vi "Read Logs.vi"() -> ()   [LabVIEW 2020]
panel:
  in  "Voltage Godograph Range":dbl caption="Amplitude Range, V" min=1.0 max=1000.0 step=1.0
  in  "Current Godograph Range":dbl caption="Amplitude Range, A" min=1.0 max=200.0 step=1.0
  in  "Voltage Amplitude Range":dbl caption="Amplitude Range, V" min=1.0 max=1000.0 step=1.0
  in  "Current Amplitude Range":dbl caption="Amplitude Range, A" min=1.0 max=200.0 step=1.0
  in  "Level Lower Limit, Cur":dbl caption="Level Lower Limit, dB" min=-200.0 max=-10.0 step=10.0
  in  "Freq Lower Limit, Cur":dbl caption="Freq Lower Limit, Hz" min=0.0 step=1.0
  in  "Freq Upper Limit, Cur":dbl caption="Freq Upper Limit, Hz" min=0.0 step=1.0
  out "Current Godograph store":cluster{"Y":dbl[], "Y":dbl[]}[](array[cluster])
  out "Voltage Godograph store":cluster{"Y":dbl[], "Y":dbl[]}[](array[cluster])
  out "Current Park Spectrum store":waveform(dbl)[](array[waveform])
  out "Voltage Park Spectrum store":waveform(dbl)[](array[waveform])
  out "Current Spectrum store":waveform(dbl)[](array[waveform])
  out "Voltage Spectrum store":waveform(dbl)[](array[waveform])
  out "Voltage store":waveform(dbl)[](array[waveform])
  out "Current store":waveform(dbl)[](array[waveform])
  in  "Hold":bool
  in  "Plot Selector":u16(ring) items=["Current", "Voltage", "Current Godograph", "Voltage Godograph", "Current Spectrum", "Voltage Spectrum", "Current Park Spectrum", "Voltage Park Spectrum"]
  in  "Choose file":bool
  out "Current Godograph":cluster{"Y":dbl[], "Y":dbl[]}[](graph)
  out "Voltage Godograph":cluster{"Y":dbl[], "Y":dbl[]}[](graph)
  out "Voltage Park Spectrum":waveform(dbl)[](graph)
  out "Current Park Spectrum":waveform(dbl)[](graph)
  out "Current Spectrum":waveform(dbl)[](graph)
  out "Voltage Spectrum":waveform(dbl)[](graph)
  out "Current":waveform(dbl)[](graph)
  out "Voltage":waveform(dbl)[](graph)
  out "error out":errorcluster
types:
  T1 = enum16{"Always On", "Always Off", "Off While Running"}
  T2 = typedef "LVPositionTypeDef.ctl" = cluster{"Left":i32, "Top":i32}
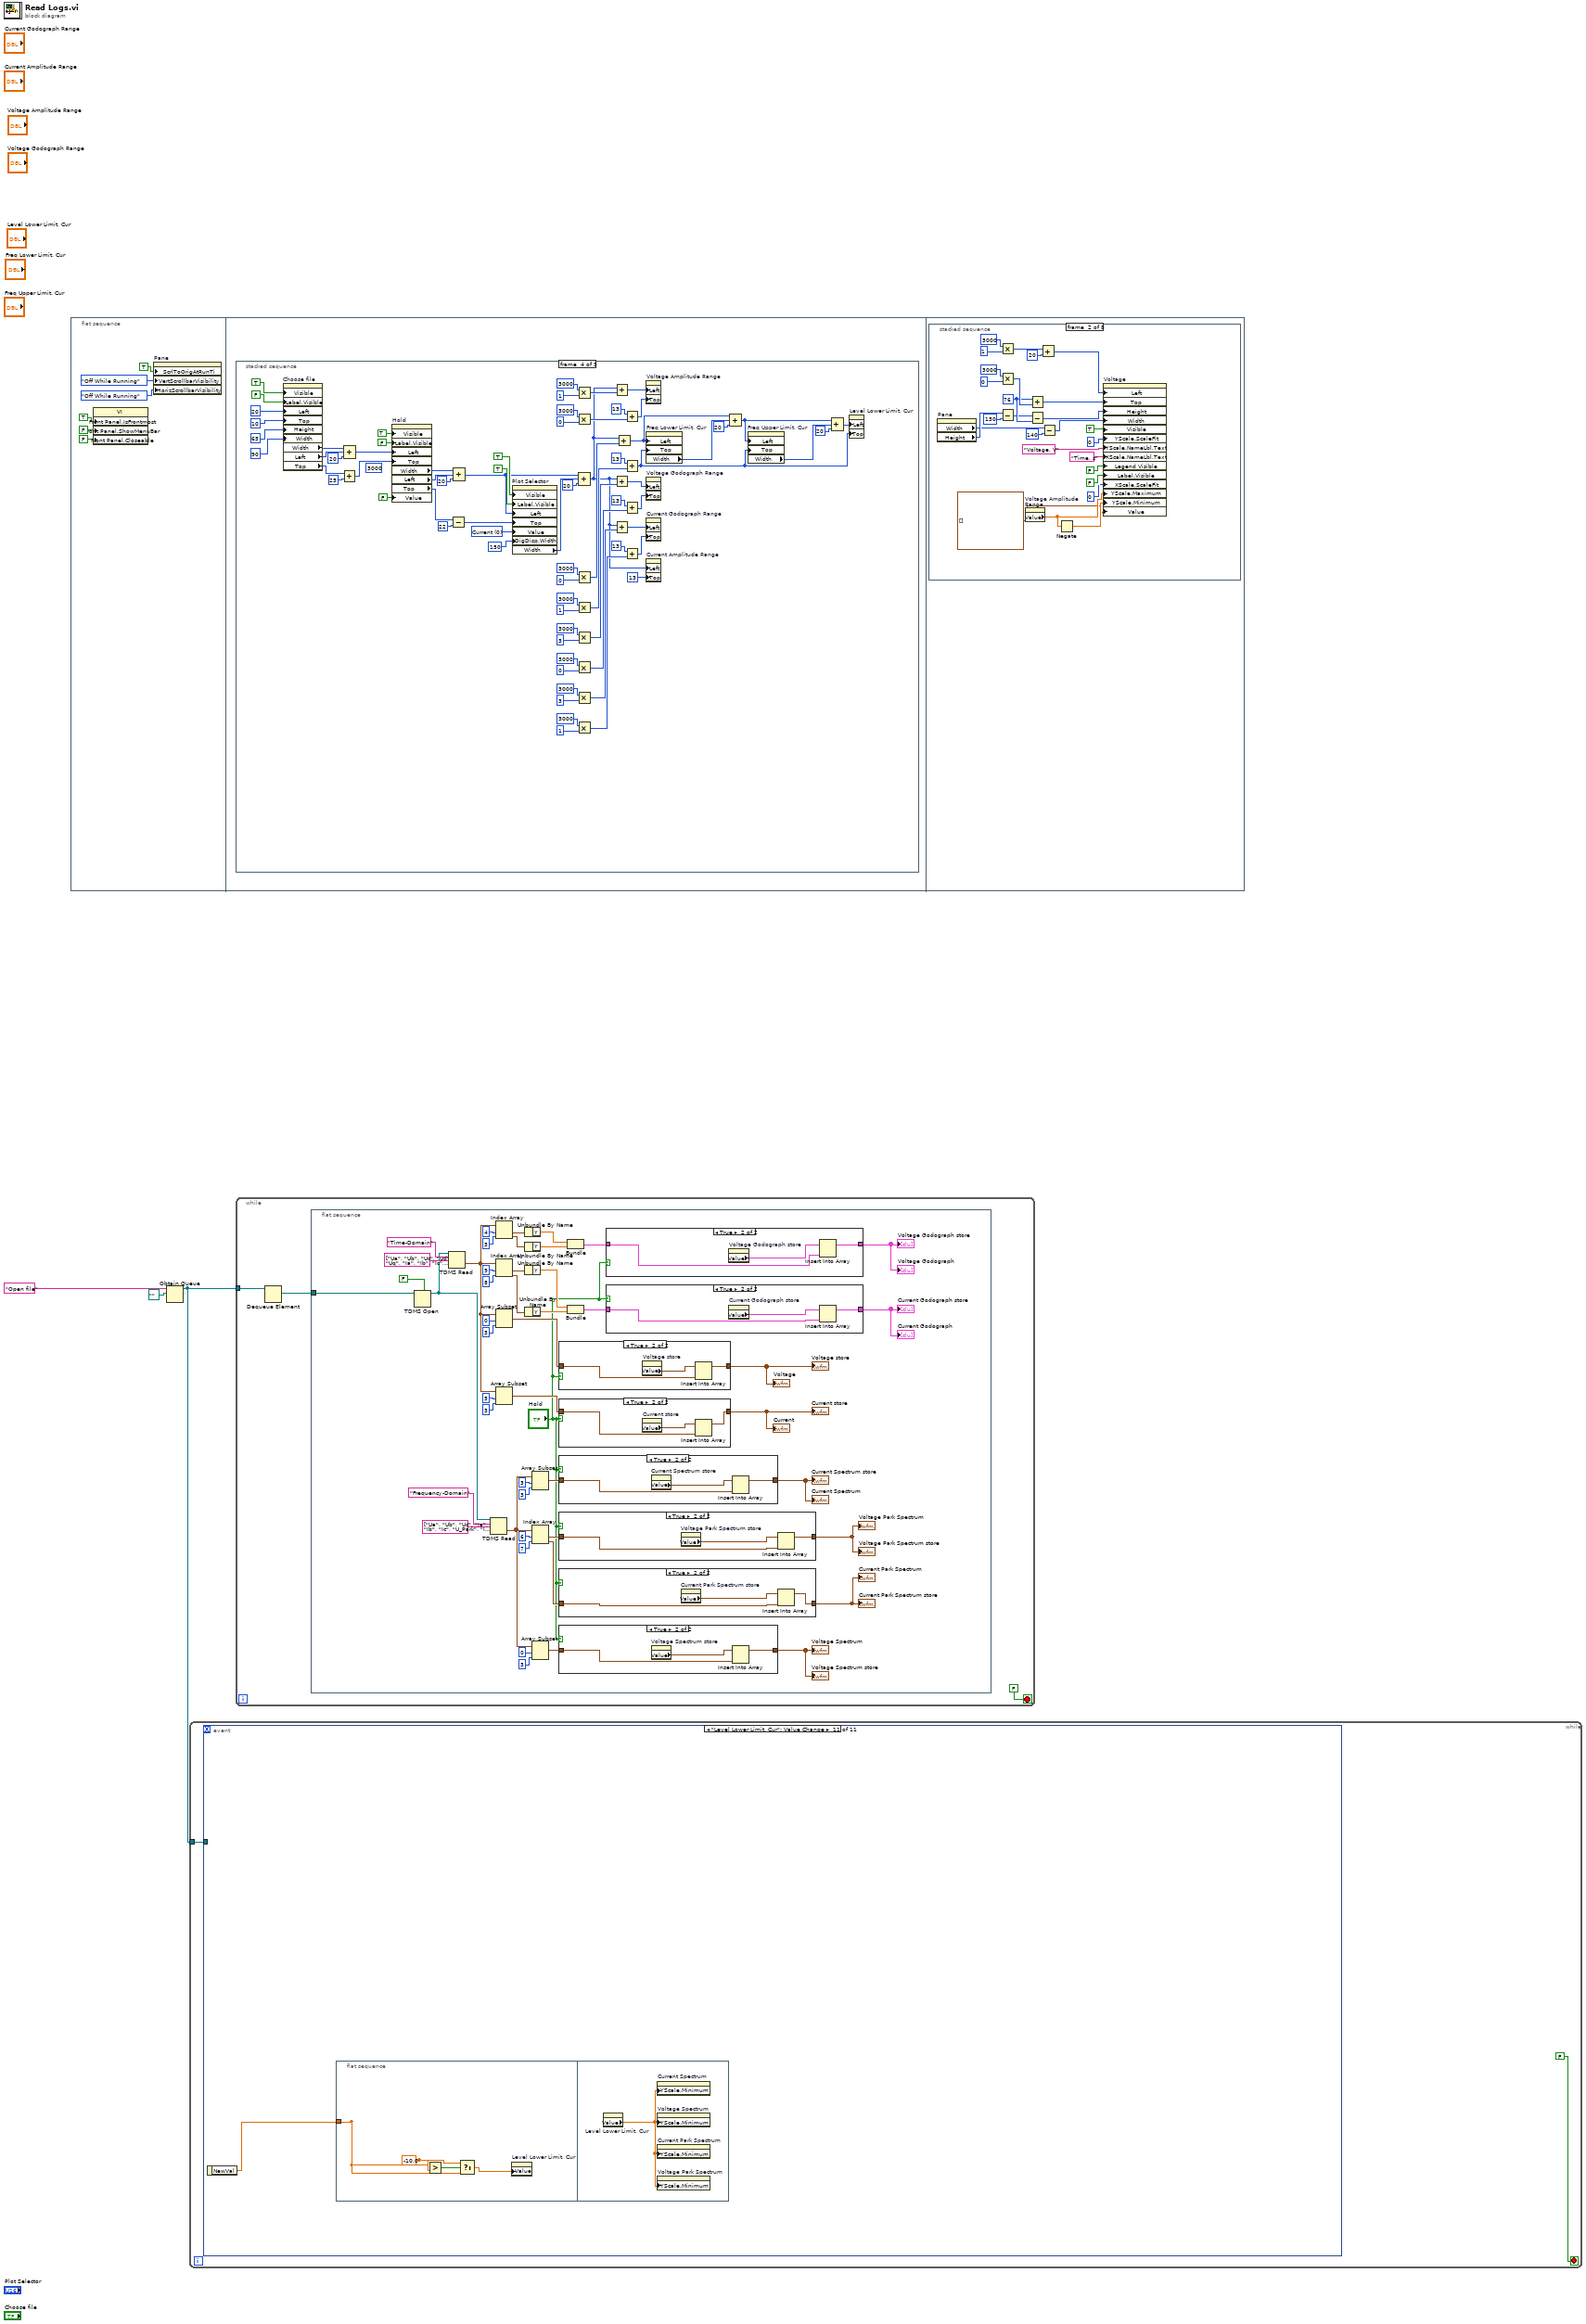
[diagram p0: block diagram]
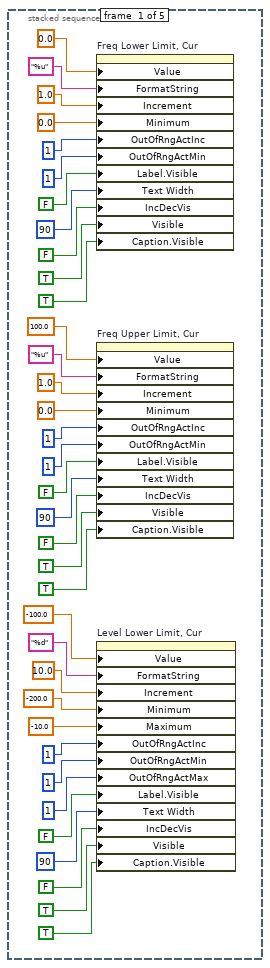
[diagram p2: hidden frame]
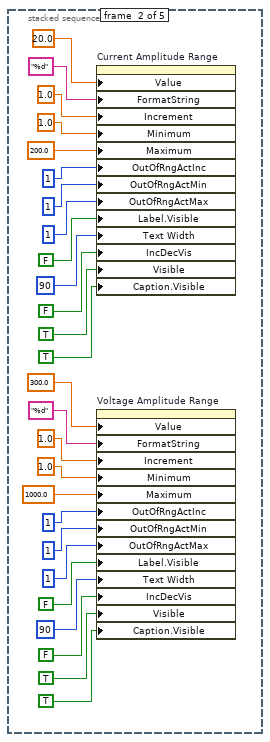
[diagram p3: hidden frame]
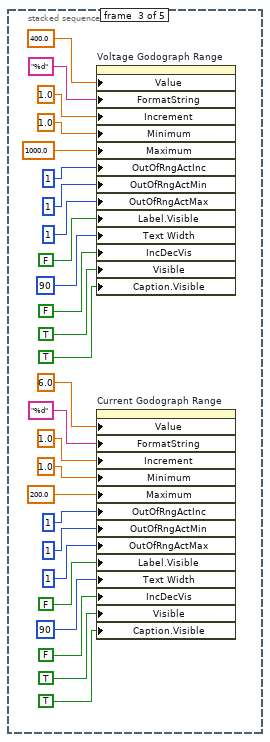
[diagram p4: hidden frame]
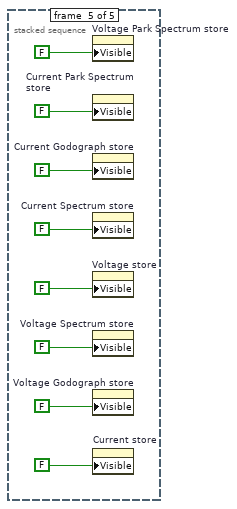
[diagram p5: hidden frame]
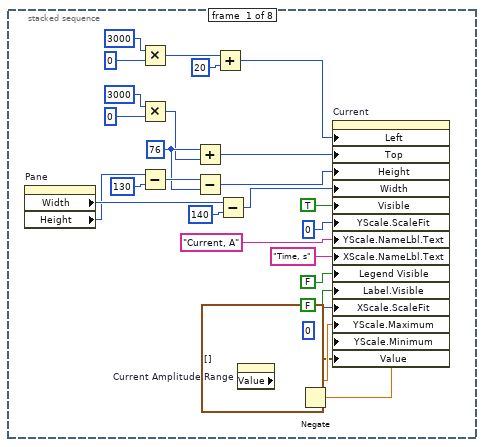
[diagram p6: hidden frame]
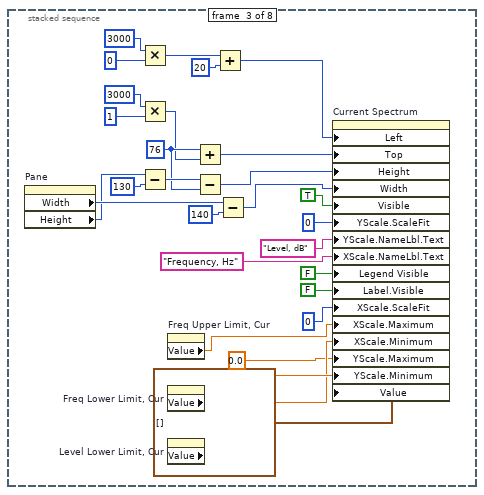
[diagram p7: hidden frame]
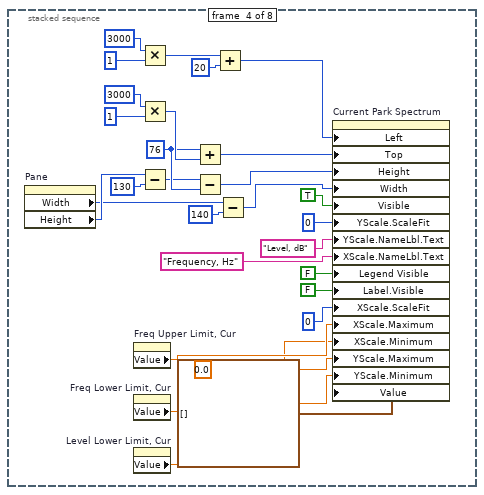
[diagram p8: hidden frame]
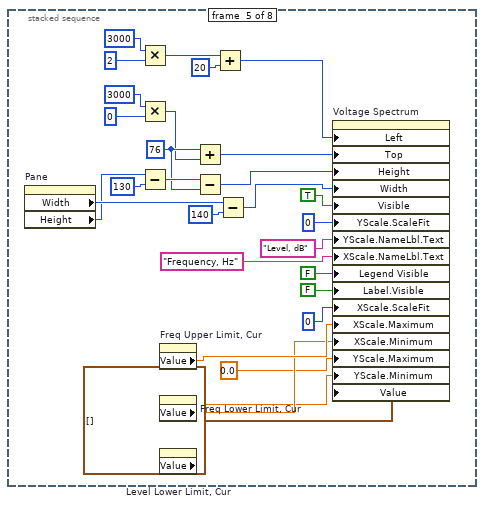
[diagram p9: hidden frame]
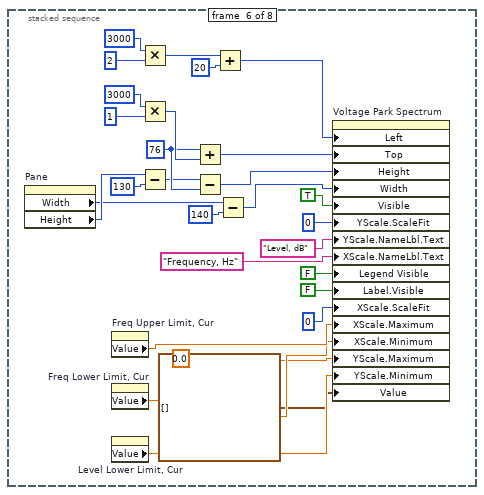
[diagram p10: hidden frame]
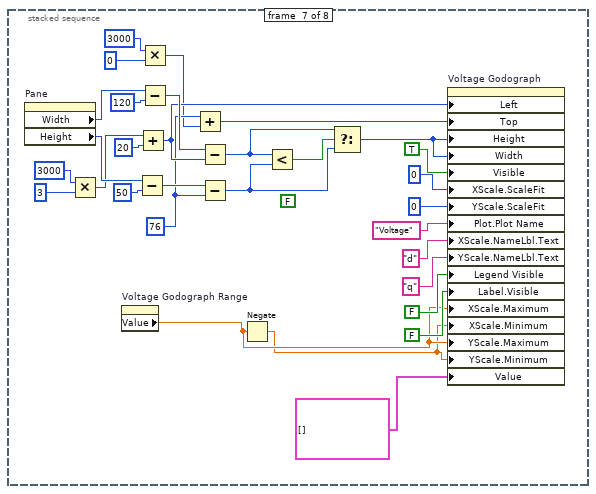
[diagram p11: hidden frame]
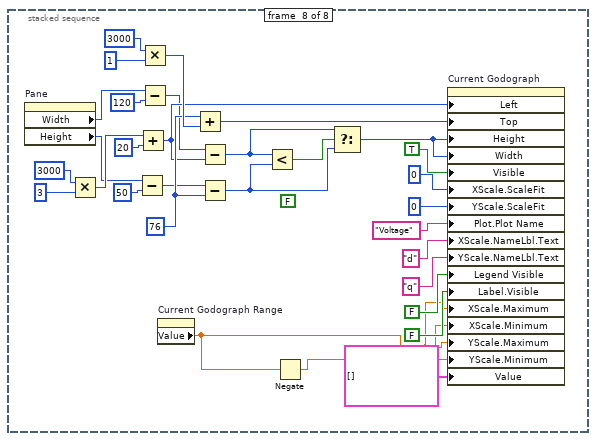
[diagram p12: hidden frame]
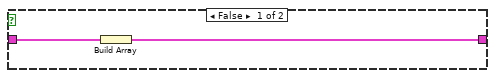
[diagram p13: hidden frame]
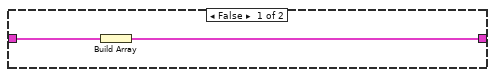
[diagram p14: hidden frame]
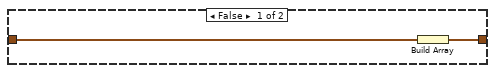
[diagram p15: hidden frame]
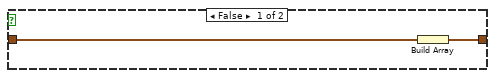
[diagram p16: hidden frame]
diagram:
  n1 = flat-sequence {
    frame #0 {
      n2 = property class="VI"("Front Panel.IsFrontmost"=TRUE ("Front Panel Window:Is Frontmost"), "Front Panel.ShowMenuBar"=FALSE ("Front Panel Window:Show Menu Bar"), "Front Panel.Closeable"=FALSE ("Front Panel Window:Closeable")) -> ()  [unwired: 2 in, 2 out]
      n3 = property on="Pane" class="Pane"("ScrlToOrigAtRunTi"=TRUE ("Scroll To Origin At Run Time"), "VertScrollbarVisibility"=T1."Off While Running" ("Vertical Scrollbar Visibility"), "HorizScrollbarVisibility"=T1."Off While Running" ("Horizontal Scrollbar Visibility")) -> ()  [unwired: 2 in, 2 out]
    }
    frame #1 {
      n4 = stacked-sequence {
        frame #0 {
          n5 = property on="Freq Lower Limit, Cur" class="DigNum (strict)"("Value"=0.0 ("Lower Limit"), "FormatString"="%u" ("Format String"), "Increment"=1.0 ("Data Entry Limits:Increment"), "Minimum"=0.0 ("Data Entry Limits:Minimum"), "OutOfRngActInc"=u8 1 ("Response to Value Outside Limits:Increment"), "OutOfRngActMin"=u8 1 ("Response to Value Outside Limits:Minimum"), "Label.Visible"=FALSE, "Text Width"=u32 90, "IncDecVis"=FALSE ("Increment/Decrement Visible?"), "Visible"=TRUE, "Caption.Visible"=TRUE) -> ()  [unwired: 2 in, 2 out]
          n6 = property on="Freq Upper Limit, Cur" class="DigNum (strict)"("Value"=100.0 ("Lower Limit"), "FormatString"="%u" ("Format String"), "Increment"=1.0 ("Data Entry Limits:Increment"), "Minimum"=0.0 ("Data Entry Limits:Minimum"), "OutOfRngActInc"=u8 1 ("Response to Value Outside Limits:Increment"), "OutOfRngActMin"=u8 1 ("Response to Value Outside Limits:Minimum"), "Label.Visible"=FALSE, "Text Width"=u32 90, "IncDecVis"=FALSE ("Increment/Decrement Visible?"), "Visible"=TRUE, "Caption.Visible"=TRUE) -> ()  [unwired: 2 in, 2 out]
          n7 = property on="Level Lower Limit, Cur" class="DigNum (strict)"("Value"=-100.0 ("Lower Limit"), "FormatString"="%d" ("Format String"), "Increment"=10.0 ("Data Entry Limits:Increment"), "Minimum"=-200.0 ("Data Entry Limits:Minimum"), "Maximum"=-10.0 ("Data Entry Limits:Maximum"), "OutOfRngActInc"=u8 1 ("Response to Value Outside Limits:Increment"), "OutOfRngActMin"=u8 1 ("Response to Value Outside Limits:Minimum"), "OutOfRngActMax"=u8 1 ("Response to Value Outside Limits:Maximum"), "Label.Visible"=FALSE, "Text Width"=u32 90, "IncDecVis"=FALSE ("Increment/Decrement Visible?"), "Visible"=TRUE, "Caption.Visible"=TRUE) -> ()  [unwired: 2 in, 2 out]
        }
        frame #1 {
          n8 = property on="Current Amplitude Range" class="DigNum (strict)"("Value"=20.0 ("Lower Limit"), "FormatString"="%d" ("Format String"), "Increment"=1.0 ("Data Entry Limits:Increment"), "Minimum"=1.0 ("Data Entry Limits:Minimum"), "Maximum"=200.0 ("Data Entry Limits:Maximum"), "OutOfRngActInc"=u8 1 ("Response to Value Outside Limits:Increment"), "OutOfRngActMin"=u8 1 ("Response to Value Outside Limits:Minimum"), "OutOfRngActMax"=u8 1 ("Response to Value Outside Limits:Maximum"), "Label.Visible"=FALSE, "Text Width"=u32 90, "IncDecVis"=FALSE ("Increment/Decrement Visible?"), "Visible"=TRUE, "Caption.Visible"=TRUE) -> ()  [unwired: 2 in, 2 out]
          n9 = property on="Voltage Amplitude Range" class="DigNum (strict)"("Value"=300.0 ("Lower Limit"), "FormatString"="%d" ("Format String"), "Increment"=1.0 ("Data Entry Limits:Increment"), "Minimum"=1.0 ("Data Entry Limits:Minimum"), "Maximum"=1000.0 ("Data Entry Limits:Maximum"), "OutOfRngActInc"=u8 1 ("Response to Value Outside Limits:Increment"), "OutOfRngActMin"=u8 1 ("Response to Value Outside Limits:Minimum"), "OutOfRngActMax"=u8 1 ("Response to Value Outside Limits:Maximum"), "Label.Visible"=FALSE, "Text Width"=u32 90, "IncDecVis"=FALSE ("Increment/Decrement Visible?"), "Visible"=TRUE, "Caption.Visible"=TRUE) -> ()  [unwired: 2 in, 2 out]
        }
        frame #2 {
          n10 = property on="Voltage Godograph Range" class="DigNum (strict)"("Value"=400.0 ("Lower Limit"), "FormatString"="%d" ("Format String"), "Increment"=1.0 ("Data Entry Limits:Increment"), "Minimum"=1.0 ("Data Entry Limits:Minimum"), "Maximum"=1000.0 ("Data Entry Limits:Maximum"), "OutOfRngActInc"=u8 1 ("Response to Value Outside Limits:Increment"), "OutOfRngActMin"=u8 1 ("Response to Value Outside Limits:Minimum"), "OutOfRngActMax"=u8 1 ("Response to Value Outside Limits:Maximum"), "Label.Visible"=FALSE, "Text Width"=u32 90, "IncDecVis"=FALSE ("Increment/Decrement Visible?"), "Visible"=TRUE, "Caption.Visible"=TRUE) -> ()  [unwired: 2 in, 2 out]
          n11 = property on="Current Godograph Range" class="DigNum (strict)"("Value"=6.0 ("Lower Limit"), "FormatString"="%d" ("Format String"), "Increment"=1.0 ("Data Entry Limits:Increment"), "Minimum"=1.0 ("Data Entry Limits:Minimum"), "Maximum"=200.0 ("Data Entry Limits:Maximum"), "OutOfRngActInc"=u8 1 ("Response to Value Outside Limits:Increment"), "OutOfRngActMin"=u8 1 ("Response to Value Outside Limits:Minimum"), "OutOfRngActMax"=u8 1 ("Response to Value Outside Limits:Maximum"), "Label.Visible"=FALSE, "Text Width"=u32 90, "IncDecVis"=FALSE ("Increment/Decrement Visible?"), "Visible"=TRUE, "Caption.Visible"=TRUE) -> ()  [unwired: 2 in, 2 out]
        }
        frame #3 {
          (unwired) 3000 ("Position:Top")
          w146 = u16 0 items=["Current", "Voltage", "Current Godograph", "Voltage Godograph", "Current Spectrum", "Voltage Spectrum", "Current Park Spectrum", "Voltage Park Spectrum"] ("Plot Selector")
          n12 = property on="Choose file" class="Bool (strict)"("Visible"=TRUE, "Label.Visible"=FALSE, "Left"=20 ("Position:Left"), "Top"=10 ("Position:Top"), "Height"=u32 65 ("Button Size:Height"), "Width"=u32 90 ("Button Size:Width")) -> ("Width"=w157:u32, "Left"=w156:i32, "Top"=w152:i32)  [unwired: 2 in, 2 out]
          n13 = Add(x=w152, y=25) -> (x+y=w150:i32)
          n14 = Compound Arithmetic op=ADD(w157, w156, 20 ("value")) -> (w155:u32)
          n15 = property on="Hold" class="Bool (strict)"("Visible"=TRUE, "Label.Visible"=FALSE, "Left"=w155, "Top"=w150, "Value"=FALSE ("Hold")) -> ("Width"=w154:u32, "Left"=w153:i32, "Top"=w149:i32)  [unwired: 2 in, 2 out]
          n16 = Subtract(x=w149, y=22) -> (x-y=w147:i32)
          n17 = Compound Arithmetic op=ADD(w154, w153, 20 ("value")) -> (w143:u32)
          n18 = property on="Plot Selector" class="Ring (strict)"("Visible"=TRUE, "Label.Visible"=TRUE, "Left"=w143, "Top"=w147, "Value"=w146, "DigDisp.Width"=u32 150 ("Digital Display.Size:Width")) -> ("Width"=w142:u32)  [unwired: 2 in, 2 out]
          n19 = Multiply(x=3000 ("Position:Top"), y=1) -> (x*y=w140:i32)
          n20 = Multiply(x=3000 ("Position:Top"), y=0) -> (x*y=w135:i32)
          n21 = Multiply(x=3000 ("Position:Top"), y=0) -> (x*y=w125:i32)
          n22 = Multiply(x=3000 ("Position:Top"), y=1) -> (x*y=w130:i32)
          n23 = Multiply(x=3000 ("Position:Top"), y=3) -> (x*y=w116:i32)
          n24 = Multiply(x=3000 ("Position:Top"), y=0) -> (x*y=w121:i32)
          n25 = Multiply(x=3000, y=3) -> (x*y=w115:i32)
          n26 = Multiply(x=3000 ("Position:Top"), y=1) -> (x*y=w111:i32)
          n27 = Compound Arithmetic op=ADD(w143, w142, u32 20 ("value")) -> (w107:u32)
          n28 = Add(x=w107, y=w140) -> (x+y=w132:u32)
          n29 = Add(x=w107, y=w116) -> (x+y=w124:u32)
          n30 = Add(x=w107, y=w115) -> (x+y=w108:u32)
          n31 = Add(x=w107, y=w125) -> (x+y=w105:u32)
          n32 = Add(x=13 ("Position:Top"), y=w135) -> (x+y=w133:i32)
          n33 = Add(x=13 ("Position:Top"), y=w130) -> (x+y=w98:i32)
          n34 = Add(x=13 ("Position:Top"), y=w121) -> (x+y=w123:i32)
          n35 = Add(x=13 ("Position:Top"), y=w111) -> (x+y=w109:i32)
          n36 = property on="Voltage Amplitude Range" class="DigNum (strict)"("Left"=w132, "Top"=w133) -> ()  [unwired: 2 in, 2 out]
          n37 = property on="Freq Lower Limit, Cur" class="DigNum (strict)"("Left"=w105, "Top"=w98) -> ("Width"=w104:u32)  [unwired: 2 in, 2 out]
          n38 = property on="Voltage Godograph Range" class="DigNum (strict)"("Left"=w124, "Top"=w123) -> ()  [unwired: 2 in, 2 out]
          n39 = property on="Current Godograph Range" class="DigNum (strict)"("Left"=w108, "Top"=w109) -> ()  [unwired: 2 in, 2 out]
          n40 = property on="Current Amplitude Range" class="DigNum (strict)"("Left"=w107, "Top"=13 ("Position:Top")) -> ()  [unwired: 2 in, 2 out]
          n41 = Compound Arithmetic op=ADD(w105, w104, u32 20 ("value")) -> (w99:u32)
          n42 = property on="Freq Upper Limit, Cur" class="DigNum (strict)"("Left"=w99, "Top"=w98) -> ("Width"=w101:u32)  [unwired: 2 in, 2 out]
          n43 = Compound Arithmetic op=ADD(w99, w101, u32 20 ("value")) -> (w100:u32)
          n44 = property on="Level Lower Limit, Cur" class="DigNum (strict)"("Left"=w100, "Top"=w98) -> ()  [unwired: 2 in, 2 out]
        }
        frame #4 {
          n45 = property on="Voltage Park Spectrum store" class="Arr (strict)"("Visible"=FALSE) -> ()  [unwired: 2 in, 2 out]
          n46 = property on="Current Park Spectrum store" class="Arr (strict)"("Visible"=FALSE) -> ()  [unwired: 2 in, 2 out]
          n47 = property on="Current Godograph store" class="Arr (strict)"("Visible"=FALSE) -> ()  [unwired: 2 in, 2 out]
          n48 = property on="Current Spectrum store" class="Arr (strict)"("Visible"=FALSE) -> ()  [unwired: 2 in, 2 out]
          n49 = property on="Voltage store" class="Arr (strict)"("Visible"=FALSE) -> ()  [unwired: 2 in, 2 out]
          n50 = property on="Voltage Spectrum store" class="Arr (strict)"("Visible"=FALSE) -> ()  [unwired: 2 in, 2 out]
          n51 = property on="Voltage Godograph store" class="Arr (strict)"("Visible"=FALSE) -> ()  [unwired: 2 in, 2 out]
          n52 = property on="Current store" class="Arr (strict)"("Visible"=FALSE) -> ()  [unwired: 2 in, 2 out]
        }
      }
    }
    frame #2 {
      n53 = stacked-sequence {
        frame #0 {
          w185 = 76 ("Position:Top")
          n54 = property on="Pane" class="Pane"() -> ("Width"=w203:u32, "Height"=w197:u32)  [unwired: 2 in, 2 out]
          n55 = Multiply(x=3000, y=0 ("Position:Left")) -> (x*y=w191:i32)
          n56 = Multiply(x=3000, y=0 ("Position:Left")) -> (x*y=w184:i32)
          n57 = Subtract(x=w197, y=u32 130) -> (x-y=w201:u32)
          n58 = Add(x=w185, y=w184) -> (x+y=w186:i32)
          n59 = Subtract(x=w201, y=w185) -> (x-y=w199:u32)
          n60 = Add(x=w191, y=20 ("Position:Left")) -> (x+y=w193:i32)
          n61 = Subtract(x=w203, y=u32 140) -> (x-y=w183:u32)
          n62 = property on="Current Amplitude Range" class="DigNum (strict)"() -> ("Value"=w180:dbl)  [unwired: 2 in, 2 out]
          n63 = Negate(x=w180) -> (-x=w179:dbl)
          n64 = property on="Current" class="WFGraph (strict)"("Left"=w193, "Top"=w186, "Height"=w199, "Width"=w183, "Visible"=TRUE, "YScale.ScaleFit"=u8 0 ("Y Scale.Scale Fit"), "YScale.NameLbl.Text"="Current, A" ("Y Scale.Name Label.Text"), "XScale.NameLbl.Text"="Time, s" ("X Scale.Name Label.Text"), "Legend Visible"=FALSE ("Legend:Visible"), "Label.Visible"=FALSE, "XScale.ScaleFit"=u8 0 ("X Scale.Scale Fit"), "YScale.Maximum"=w180, "YScale.Minimum"=w179, "Value"=waveform(dbl)[] [] ("Current")) -> ()  [unwired: 2 in, 2 out]
        }
        frame #1 {
          w230 = 76 ("Position:Top")
          n65 = property on="Pane" class="Pane"() -> ("Width"=w212:u32, "Height"=w218:u32)  [unwired: 2 in, 2 out]
          n66 = Multiply(x=3000, y=1 ("Position:Left")) -> (x*y=w224:i32)
          n67 = Multiply(x=3000, y=0 ("Position:Left")) -> (x*y=w231:i32)
          n68 = Subtract(x=w218, y=u32 130) -> (x-y=w214:u32)
          n69 = property on="Voltage Amplitude Range" class="DigNum (strict)"() -> ("Value"=w206:dbl)  [unwired: 2 in, 2 out]
          n70 = Add(x=w230, y=w231) -> (x+y=w229:i32)
          n71 = Subtract(x=w214, y=w230) -> (x-y=w216:u32)
          n72 = Add(x=w224, y=20 ("Position:Left")) -> (x+y=w222:i32)
          n73 = Subtract(x=w212, y=u32 140) -> (x-y=w210:u32)
          n74 = Negate(x=w206) -> (-x=w207:dbl)
          n75 = property on="Voltage" class="WFGraph (strict)"("Left"=w222, "Top"=w229, "Height"=w216, "Width"=w210, "Visible"=TRUE, "YScale.ScaleFit"=u8 0 ("Y Scale.Scale Fit"), "YScale.NameLbl.Text"="Voltage, V" ("Y Scale.Name Label.Text"), "XScale.NameLbl.Text"="Time, s" ("X Scale.Name Label.Text"), "Legend Visible"=FALSE ("Legend:Visible"), "Label.Visible"=FALSE, "XScale.ScaleFit"=u8 0 ("X Scale.Scale Fit"), "YScale.Maximum"=w206, "YScale.Minimum"=w207, "Value"=waveform(dbl)[] [] ("Current")) -> ()  [unwired: 2 in, 2 out]
        }
        frame #2 {
          w242 = 76 ("Position:Top")
          n76 = property on="Pane" class="Pane"() -> ("Width"=w259:u32, "Height"=w253:u32)  [unwired: 2 in, 2 out]
          n77 = Multiply(x=3000, y=0 ("Position:Left")) -> (x*y=w247:i32)
          n78 = Multiply(x=3000, y=1 ("Position:Left")) -> (x*y=w241:i32)
          n79 = Subtract(x=w253, y=u32 130) -> (x-y=w257:u32)
          n80 = property on="Freq Upper Limit, Cur" class="DigNum (strict)"() -> ("Value"=w234:dbl)  [unwired: 2 in, 2 out]
          n81 = property on="Freq Lower Limit, Cur" class="DigNum (strict)"() -> ("Value"=w235:dbl)  [unwired: 2 in, 2 out]
          n82 = property on="Level Lower Limit, Cur" class="DigNum (strict)"() -> ("Value"=w236:dbl)  [unwired: 2 in, 2 out]
          n83 = Add(x=w242, y=w241) -> (x+y=w243:i32)
          n84 = Subtract(x=w257, y=w242) -> (x-y=w255:u32)
          n85 = Add(x=w247, y=20 ("Position:Left")) -> (x+y=w249:i32)
          n86 = Subtract(x=w259, y=u32 140) -> (x-y=w239:u32)
          n87 = property on="Current Spectrum" class="WFGraph (strict)"("Left"=w249, "Top"=w243, "Height"=w255, "Width"=w239, "Visible"=TRUE, "YScale.ScaleFit"=u8 0 ("Y Scale.Scale Fit"), "YScale.NameLbl.Text"="Level, dB" ("Y Scale.Name Label.Text"), "XScale.NameLbl.Text"="Frequency, Hz" ("X Scale.Name Label.Text"), "Legend Visible"=FALSE ("Legend:Visible"), "Label.Visible"=FALSE, "XScale.ScaleFit"=u8 0 ("X Scale.Scale Fit"), "XScale.Maximum"=w234, "XScale.Minimum"=w235, "YScale.Maximum"=0.0 ("Y Scale.Range:Maximum"), "YScale.Minimum"=w236, "Value"=waveform(dbl)[] [] ("Current")) -> ()  [unwired: 2 in, 2 out]
        }
        frame #3 {
          w287 = 76 ("Position:Top")
          n88 = property on="Pane" class="Pane"() -> ("Width"=w270:u32, "Height"=w276:u32)  [unwired: 2 in, 2 out]
          n89 = property on="Freq Upper Limit, Cur" class="DigNum (strict)"() -> ("Value"=w265:dbl)  [unwired: 2 in, 2 out]
          n90 = property on="Freq Lower Limit, Cur" class="DigNum (strict)"() -> ("Value"=w264:dbl)  [unwired: 2 in, 2 out]
          n91 = property on="Level Lower Limit, Cur" class="DigNum (strict)"() -> ("Value"=w262:dbl)  [unwired: 2 in, 2 out]
          n92 = Multiply(x=3000, y=1 ("Position:Left")) -> (x*y=w282:i32)
          n93 = Multiply(x=3000, y=1 ("Position:Left")) -> (x*y=w288:i32)
          n94 = Subtract(x=w276, y=u32 130) -> (x-y=w272:u32)
          n95 = Add(x=w287, y=w288) -> (x+y=w286:i32)
          n96 = Subtract(x=w272, y=w287) -> (x-y=w274:u32)
          n97 = Add(x=w282, y=20 ("Position:Left")) -> (x+y=w280:i32)
          n98 = Subtract(x=w270, y=u32 140) -> (x-y=w268:u32)
          n99 = property on="Current Park Spectrum" class="WFGraph (strict)"("Left"=w280, "Top"=w286, "Height"=w274, "Width"=w268, "Visible"=TRUE, "YScale.ScaleFit"=u8 0 ("Y Scale.Scale Fit"), "YScale.NameLbl.Text"="Level, dB" ("Y Scale.Name Label.Text"), "XScale.NameLbl.Text"="Frequency, Hz" ("X Scale.Name Label.Text"), "Legend Visible"=FALSE ("Legend:Visible"), "Label.Visible"=FALSE, "XScale.ScaleFit"=u8 0 ("X Scale.Scale Fit"), "XScale.Maximum"=w265, "XScale.Minimum"=w264, "YScale.Maximum"=0.0 ("Y Scale.Range:Maximum"), "YScale.Minimum"=w262, "Value"=waveform(dbl)[] [] ("Current")) -> ()  [unwired: 2 in, 2 out]
        }
        frame #4 {
          w300 = 76 ("Position:Top")
          n100 = property on="Pane" class="Pane"() -> ("Width"=w317:u32, "Height"=w311:u32)  [unwired: 2 in, 2 out]
          n101 = Multiply(x=3000, y=2 ("Position:Left")) -> (x*y=w305:i32)
          n102 = Multiply(x=3000, y=0 ("Position:Left")) -> (x*y=w299:i32)
          n103 = Subtract(x=w311, y=u32 130) -> (x-y=w315:u32)
          n104 = property on="Freq Upper Limit, Cur" class="DigNum (strict)"() -> ("Value"=w294:dbl)  [unwired: 2 in, 2 out]
          n105 = property on="Freq Lower Limit, Cur" class="DigNum (strict)"() -> ("Value"=w293:dbl)  [unwired: 2 in, 2 out]
          n106 = property on="Level Lower Limit, Cur" class="DigNum (strict)"() -> ("Value"=w291:dbl)  [unwired: 2 in, 2 out]
          n107 = Add(x=w300, y=w299) -> (x+y=w301:i32)
          n108 = Subtract(x=w315, y=w300) -> (x-y=w313:u32)
          n109 = Add(x=w305, y=20 ("Position:Left")) -> (x+y=w307:i32)
          n110 = Subtract(x=w317, y=u32 140) -> (x-y=w297:u32)
          n111 = property on="Voltage Spectrum" class="WFGraph (strict)"("Left"=w307, "Top"=w301, "Height"=w313, "Width"=w297, "Visible"=TRUE, "YScale.ScaleFit"=u8 0 ("Y Scale.Scale Fit"), "YScale.NameLbl.Text"="Level, dB" ("Y Scale.Name Label.Text"), "XScale.NameLbl.Text"="Frequency, Hz" ("X Scale.Name Label.Text"), "Legend Visible"=FALSE ("Legend:Visible"), "Label.Visible"=FALSE, "XScale.ScaleFit"=u8 0 ("X Scale.Scale Fit"), "XScale.Maximum"=w294, "XScale.Minimum"=w293, "YScale.Maximum"=0.0 ("Y Scale.Range:Maximum"), "YScale.Minimum"=w291, "Value"=waveform(dbl)[] [] ("Current")) -> ()  [unwired: 2 in, 2 out]
        }
        frame #5 {
          w345 = 76 ("Position:Top")
          n112 = property on="Pane" class="Pane"() -> ("Width"=w328:u32, "Height"=w334:u32)  [unwired: 2 in, 2 out]
          n113 = property on="Freq Upper Limit, Cur" class="DigNum (strict)"() -> ("Value"=w323:dbl)  [unwired: 2 in, 2 out]
          n114 = property on="Freq Lower Limit, Cur" class="DigNum (strict)"() -> ("Value"=w322:dbl)  [unwired: 2 in, 2 out]
          n115 = property on="Level Lower Limit, Cur" class="DigNum (strict)"() -> ("Value"=w320:dbl)  [unwired: 2 in, 2 out]
          n116 = Multiply(x=3000, y=2 ("Position:Left")) -> (x*y=w340:i32)
          n117 = Multiply(x=3000, y=1 ("Position:Left")) -> (x*y=w346:i32)
          n118 = Subtract(x=w334, y=u32 130) -> (x-y=w330:u32)
          n119 = Add(x=w345, y=w346) -> (x+y=w344:i32)
          n120 = Subtract(x=w330, y=w345) -> (x-y=w332:u32)
          n121 = Add(x=w340, y=20 ("Position:Left")) -> (x+y=w338:i32)
          n122 = Subtract(x=w328, y=u32 140) -> (x-y=w326:u32)
          n123 = property on="Voltage Park Spectrum" class="WFGraph (strict)"("Left"=w338, "Top"=w344, "Height"=w332, "Width"=w326, "Visible"=TRUE, "YScale.ScaleFit"=u8 0 ("Y Scale.Scale Fit"), "YScale.NameLbl.Text"="Level, dB" ("Y Scale.Name Label.Text"), "XScale.NameLbl.Text"="Frequency, Hz" ("X Scale.Name Label.Text"), "Legend Visible"=FALSE ("Legend:Visible"), "Label.Visible"=FALSE, "XScale.ScaleFit"=u8 0 ("X Scale.Scale Fit"), "XScale.Maximum"=w323, "XScale.Minimum"=w322, "YScale.Maximum"=0.0 ("Y Scale.Range:Maximum"), "YScale.Minimum"=w320, "Value"=waveform(dbl)[] [] ("Current")) -> ()  [unwired: 2 in, 2 out]
        }
        frame #6 {
          (unwired) FALSE ("Visible")
          w353 = 76 ("Position:Top")
          n124 = property on="Pane" class="Pane"() -> ("Width"=w372:u32, "Height"=w369:u32)  [unwired: 2 in, 2 out]
          n125 = Multiply(x=3000, y=3 ("Position:Left")) -> (x*y=w356:i32)
          n126 = property on="Voltage Godograph Range" class="DigNum (strict)"() -> ("Value"=w350:dbl)  [unwired: 2 in, 2 out]
          n127 = Subtract(x=w369, y=u32 50) -> (x-y=w375:u32)
          n128 = Add(x=w356, y=20 ("value")) -> (x+y=w364:i32)
          n129 = Multiply(x=3000, y=0 ("Position:Left")) -> (x*y=w352:i32)
          n130 = Subtract(x=w372, y=u32 120) -> (x-y=w376:u32)
          n131 = Add(x=w353, y=w352) -> (x+y=w351:i32)
          n132 = Subtract(x=w376, y=w364) -> (x-y=w370:u32)
          n133 = Subtract(x=w375, y=w353) -> (x-y=w368:u32)
          n134 = Negate(x=w350) -> (-x=w349:dbl)
          n135 = Less?(x=w370, y=w368) -> (x < y?=w373:bool)
          n136 = Select(t=w370, s=w373, f=w368) -> (s? t:f=w371:u32)
          n137 = property on="Voltage Godograph" class="XYGraph (strict)"("Left"=w364, "Top"=w351, "Height"=w371, "Width"=w371, "Visible"=TRUE, "XScale.ScaleFit"=u8 0 ("X Scale.Scale Fit"), "YScale.ScaleFit"=u8 0 ("Y Scale.Scale Fit"), "Plot.Plot Name"="Voltage", "XScale.NameLbl.Text"="d" ("X Scale.Name Label.Text"), "YScale.NameLbl.Text"="q" ("Y Scale.Name Label.Text"), "Legend Visible"=FALSE ("Legend:Visible"), "Label.Visible"=FALSE, "XScale.Maximum"=w350, "XScale.Minimum"=w349, "YScale.Maximum"=w350, "YScale.Minimum"=w349, "Value"=cluster{"Y":dbl[], "Y":dbl[]}[] [] ("Current Godograph")) -> ()  [unwired: 2 in, 2 out]
        }
        frame #7 {
          (unwired) FALSE ("Visible")
          w407 = 76 ("Position:Top")
          n138 = property on="Pane" class="Pane"() -> ("Width"=w388:u32, "Height"=w391:u32)  [unwired: 2 in, 2 out]
          n139 = Multiply(x=3000, y=3 ("Position:Left")) -> (x*y=w404:i32)
          n140 = Subtract(x=w391, y=u32 50) -> (x-y=w385:u32)
          n141 = Add(x=w404, y=20 ("value")) -> (x+y=w396:i32)
          n142 = Multiply(x=3000, y=1 ("Position:Left")) -> (x*y=w408:i32)
          n143 = Subtract(x=w388, y=u32 120) -> (x-y=w384:u32)
          n144 = property on="Current Godograph Range" class="DigNum (strict)"() -> ("Value"=w381:dbl)  [unwired: 2 in, 2 out]
          n145 = Add(x=w407, y=w408) -> (x+y=w409:i32)
          n146 = Subtract(x=w384, y=w396) -> (x-y=w390:u32)
          n147 = Subtract(x=w385, y=w407) -> (x-y=w392:u32)
          n148 = Less?(x=w390, y=w392) -> (x < y?=w387:bool)
          n149 = Negate(x=w381) -> (-x=w380:dbl)
          n150 = Select(t=w390, s=w387, f=w392) -> (s? t:f=w389:u32)
          n151 = property on="Current Godograph" class="XYGraph (strict)"("Left"=w396, "Top"=w409, "Height"=w389, "Width"=w389, "Visible"=TRUE, "XScale.ScaleFit"=u8 0 ("X Scale.Scale Fit"), "YScale.ScaleFit"=u8 0 ("Y Scale.Scale Fit"), "Plot.Plot Name"="Voltage", "XScale.NameLbl.Text"="d" ("X Scale.Name Label.Text"), "YScale.NameLbl.Text"="q" ("Y Scale.Name Label.Text"), "Legend Visible"=FALSE ("Legend:Visible"), "Label.Visible"=FALSE, "XScale.Maximum"=w381, "XScale.Minimum"=w380, "YScale.Maximum"=w381, "YScale.Minimum"=w380, "Value"=cluster{"Y":dbl[], "Y":dbl[]}[] [] ("Current Godograph")) -> ()  [unwired: 2 in, 2 out]
        }
      }
    }
  }
  n152 = Obtain Queue(name (unnamed)="Open file", element data type=path "") -> (queue out=w1:refnum<queue>)  [unwired: 3 in, 2 out]
  n153 = while {
    tunnel: w1 -> [w410]
    stop <- FALSE stop-if-true
    n154 = event shown="[10] \"Level Lower Limit, Cur\": Value Change" {
      selector: _ -> [_ _ _ _ _ _ _ _ _ _ _]
      dyn-events: _ -> [_ _ _ _ _ _ _ _ _ _ _]
      timeout: _ -> [_ _ _ _ _ _ _ _ _ _ _]
      tunnel: w410 -> [_ w413 _ _ _ _ _ _ _ _ _]
      event Timeout {
        n155 = event-data() -> ()  [unwired: 1 in, 3 out]
      }
      event "Choose file": Value Change {
        n156 = event-data() -> ("CtlRef"=w412:refnum<vi>)  [unwired: 1 in, 5 out]
        n157 = property on="Property Node" class="Bool (strict)"(reference=w412, "Value"=FALSE ("Choose file")) -> ()  [unwired: 1 in, 2 out]
        n158 = call "File Dialog"("pattern (all files)"="*.tdms") -> ("selected path"=w414:path, "cancelled"=w415:bool, "error out"=→"error out":errorcluster)  [unwired: 11 in, 1 out]
        n159 = case shown="False" w415 {
          tunnel: w414 -> [w419 _]
          tunnel: w413 -> [w420 _]
          frame False {
            n160 = Enqueue Element(queue=w420, element=w419) -> ()  [unwired: 2 in, 3 out]
          }
          frame True {
          }
        }
      }
      event Key Down {
        n161 = event-data() -> ("Char"=w422:i16, "PlatMods.Ctrl"=w421:bool)  [unwired: 1 in]
        n162 = case shown="True" w421 {
          tunnel: w422 -> [_ w425]
          frame False {
          }
          frame True {
            n163 = Subtract(x=w425, y=i16 49) -> (x-y=w423:i16)
            n164 = case shown="7" w423 {
              selector: w423 -> [_ w428 w455 w484 w513 w553 w591 w629 w667]
              frame Default {
              }
              frame 0 {
                n165 = property on="Current" class="WFGraph (strict)"() -> ("Position"=w451:T2)  [unwired: 2 in, 2 out]
                n166 = Unbundle By Name(w451) -> ("Left"=w450:i32, "Top"=w449:i32)
                n167 = Subtract(x=w450, y=20) -> (x-y=w430:i32)
                n168 = Subtract(x=w449, y=76) -> (x-y=w429:i32)
                n169 = Bundle By Name(cluster=w451, "Left"=w430, "Top"=w429) -> (w452:T2)
                n170 = Add(x=w430, y=20 ("Position:Left")) -> (x+y=w432:i32)
                n171 = Add(x=w429, y=10 ("Position:Top")) -> (x+y=w431:i32)
                n172 = property on="Pane" class="Pane"("Origin"=w452) -> ()  [unwired: 2 in, 2 out]
                n173 = property on="Choose file" class="Bool (strict)"("Left"=w432, "Top"=w431, "Height"=u32 65 ("Button Size:Height"), "Width"=u32 90 ("Button Size:Width")) -> ("Width"=w444:u32, "Left"=w443:i32, "Top"=w439:i32)  [unwired: 2 in, 2 out]
                n174 = Add(x=w439, y=25) -> (x+y=w437:i32)
                n175 = Compound Arithmetic op=ADD(w444, w443, 20 ("value")) -> (w442:u32)
                n176 = property on="Hold" class="Bool (strict)"("Left"=w442, "Top"=w437) -> ("Width"=w441:u32, "Left"=w440:i32, "Top"=w436:i32)  [unwired: 2 in, 2 out]
                n177 = Subtract(x=w436, y=22) -> (x-y=w427:i32)
                n178 = Compound Arithmetic op=ADD(w441, w440, 20 ("value")) -> (w426:u32)
                n179 = property on="Plot Selector" class="Ring (strict)"("Left"=w426, "Top"=w427, "Value"=w428) -> ()  [unwired: 2 in, 2 out]
              }
              frame 1 {
                n180 = property on="Voltage" class="WFGraph (strict)"() -> ("Position"=w480:T2)  [unwired: 2 in, 2 out]
                n181 = Unbundle By Name(w480) -> ("Left"=w479:i32, "Top"=w478:i32)
                n182 = Subtract(x=w479, y=20) -> (x-y=w457:i32)
                n183 = Subtract(x=w478, y=76) -> (x-y=w456:i32)
                n184 = Bundle By Name(cluster=w480, "Left"=w457, "Top"=w456) -> (w481:T2)
                n185 = Add(x=w457, y=20 ("Position:Left")) -> (x+y=w459:i32)
                n186 = Add(x=w456, y=10 ("Position:Top")) -> (x+y=w458:i32)
                n187 = property on="Pane" class="Pane"("Origin"=w481) -> ()  [unwired: 2 in, 2 out]
                n188 = property on="Choose file" class="Bool (strict)"("Left"=w459, "Top"=w458, "Height"=u32 65 ("Button Size:Height"), "Width"=u32 90 ("Button Size:Width")) -> ("Width"=w472:u32, "Left"=w471:i32, "Top"=w467:i32)  [unwired: 2 in, 2 out]
                n189 = Add(x=w467, y=25) -> (x+y=w465:i32)
                n190 = Compound Arithmetic op=ADD(w472, w471, 20 ("value")) -> (w470:u32)
                n191 = property on="Hold" class="Bool (strict)"("Left"=w470, "Top"=w465) -> ("Width"=w469:u32, "Left"=w468:i32, "Top"=w464:i32)  [unwired: 2 in, 2 out]
                n192 = Subtract(x=w464, y=22) -> (x-y=w462:i32)
                n193 = Compound Arithmetic op=ADD(w469, w468, 20 ("value")) -> (w476:u32)
                n194 = property on="Plot Selector" class="Ring (strict)"("Left"=w476, "Top"=w462, "Value"=w455) -> ()  [unwired: 2 in, 2 out]
              }
              frame 2 {
                n195 = property on="Current Godograph" class="XYGraph (strict)"() -> ("Position"=w509:T2)  [unwired: 2 in, 2 out]
                n196 = Unbundle By Name(w509) -> ("Left"=w508:i32, "Top"=w507:i32)
                n197 = Subtract(x=w508, y=20) -> (x-y=w486:i32)
                n198 = Subtract(x=w507, y=76) -> (x-y=w485:i32)
                n199 = Bundle By Name(cluster=w509, "Left"=w486, "Top"=w485) -> (w510:T2)
                n200 = Add(x=w486, y=20 ("Position:Left")) -> (x+y=w488:i32)
                n201 = Add(x=w485, y=10 ("Position:Top")) -> (x+y=w487:i32)
                n202 = property on="Pane" class="Pane"("Origin"=w510) -> ()  [unwired: 2 in, 2 out]
                n203 = property on="Choose file" class="Bool (strict)"("Left"=w488, "Top"=w487, "Height"=u32 65 ("Button Size:Height"), "Width"=u32 90 ("Button Size:Width")) -> ("Width"=w501:u32, "Left"=w500:i32, "Top"=w496:i32)  [unwired: 2 in, 2 out]
                n204 = Add(x=w496, y=25) -> (x+y=w494:i32)
                n205 = Compound Arithmetic op=ADD(w501, w500, 20 ("value")) -> (w499:u32)
                n206 = property on="Hold" class="Bool (strict)"("Left"=w499, "Top"=w494) -> ("Width"=w498:u32, "Left"=w497:i32, "Top"=w493:i32)  [unwired: 2 in, 2 out]
                n207 = Subtract(x=w493, y=22) -> (x-y=w491:i32)
                n208 = Compound Arithmetic op=ADD(w498, w497, 20 ("value")) -> (w505:u32)
                n209 = property on="Plot Selector" class="Ring (strict)"("Left"=w505, "Top"=w491, "Value"=w484) -> ()  [unwired: 2 in, 2 out]
              }
              frame 3 {
                n210 = property on="Voltage Godograph" class="XYGraph (strict)"() -> ("Position"=w540:T2)  [unwired: 2 in, 2 out]
                n211 = Unbundle By Name(w540) -> ("Left"=w539:i32, "Top"=w538:i32)
                n212 = Subtract(x=w539, y=20) -> (x-y=w515:i32)
                n213 = Subtract(x=w538, y=76) -> (x-y=w514:i32)
                n214 = Bundle By Name(cluster=w540, "Left"=w515, "Top"=w514) -> (w541:T2)
                n215 = Add(x=w515, y=20 ("Position:Left")) -> (x+y=w517:i32)
                n216 = Add(x=w514, y=10 ("Position:Top")) -> (x+y=w516:i32)
                n217 = property on="Pane" class="Pane"("Origin"=w541) -> ()  [unwired: 2 in, 2 out]
                n218 = property on="Choose file" class="Bool (strict)"("Left"=w517, "Top"=w516, "Height"=u32 65 ("Button Size:Height"), "Width"=u32 90 ("Button Size:Width")) -> ("Width"=w530:u32, "Left"=w529:i32, "Top"=w525:i32)  [unwired: 2 in, 2 out]
                n219 = Add(x=w525, y=25) -> (x+y=w523:i32)
                n220 = Compound Arithmetic op=ADD(w530, w529, 20 ("value")) -> (w528:u32)
                n221 = property on="Hold" class="Bool (strict)"("Left"=w528, "Top"=w523) -> ("Width"=w527:u32, "Left"=w526:i32, "Top"=w522:i32)  [unwired: 2 in, 2 out]
                n222 = Subtract(x=w522, y=22) -> (x-y=w520:i32)
                n223 = Compound Arithmetic op=ADD(w527, w526, 20 ("value")) -> (w534:u32)
                n224 = property on="Plot Selector" class="Ring (strict)"("Left"=w534, "Top"=w520, "Value"=w513) -> ()  [unwired: 2 in, 2 out]
              }
              frame 4 {
                n225 = property on="Current Spectrum" class="WFGraph (strict)"() -> ("Position"=w576:T2)  [unwired: 2 in, 2 out]
                n226 = Unbundle By Name(w576) -> ("Left"=w575:i32, "Top"=w574:i32)
                n227 = Subtract(x=w575, y=20) -> (x-y=w555:i32)
                n228 = Subtract(x=w574, y=76) -> (x-y=w554:i32)
                n229 = Bundle By Name(cluster=w576, "Left"=w555, "Top"=w554) -> (w577:T2)
                n230 = Add(x=w555, y=20 ("Position:Left")) -> (x+y=w557:i32)
                n231 = Add(x=w554, y=10 ("Position:Top")) -> (x+y=w556:i32)
                n232 = property on="Pane" class="Pane"("Origin"=w577) -> ()  [unwired: 2 in, 2 out]
                n233 = property on="Choose file" class="Bool (strict)"("Left"=w557, "Top"=w556, "Height"=u32 65 ("Button Size:Height"), "Width"=u32 90 ("Button Size:Width")) -> ("Width"=w569:u32, "Left"=w568:i32, "Top"=w564:i32)  [unwired: 2 in, 2 out]
                n234 = Add(x=w564, y=25) -> (x+y=w562:i32)
                n235 = Compound Arithmetic op=ADD(w569, w568, 20 ("value")) -> (w567:u32)
                n236 = property on="Hold" class="Bool (strict)"("Left"=w567, "Top"=w562) -> ("Width"=w566:u32, "Left"=w565:i32, "Top"=w561:i32)  [unwired: 2 in, 2 out]
                n237 = Subtract(x=w561, y=22) -> (x-y=w542:i32)
                n238 = Compound Arithmetic op=ADD(w566, w565, 20 ("value")) -> (w543:u32)
                n239 = property on="Plot Selector" class="Ring (strict)"("Left"=w543, "Top"=w542, "Value"=w553) -> ("Width"=w544:u32)  [unwired: 2 in, 2 out]
                n240 = Compound Arithmetic op=ADD(w543, w544, u32 20 ("value")) -> (w552:u32)
                n241 = property on="Freq Lower Limit, Cur" class="DigNum (strict)"("Left"=w552, "Top"=w542) -> ("Width"=w545:u32)  [unwired: 2 in, 2 out]
                n242 = Compound Arithmetic op=ADD(w552, w545, u32 20 ("value")) -> (w550:u32)
                n243 = property on="Freq Upper Limit, Cur" class="DigNum (strict)"("Left"=w550, "Top"=w542) -> ("Width"=w548:u32)  [unwired: 2 in, 2 out]
                n244 = Compound Arithmetic op=ADD(w550, w548, u32 20 ("value")) -> (w549:u32)
                n245 = property on="Level Lower Limit, Cur" class="DigNum (strict)"("Left"=w549, "Top"=w542) -> ()  [unwired: 2 in, 2 out]
              }
              frame 5 {
                n246 = property on="Voltage Spectrum" class="WFGraph (strict)"() -> ("Position"=w614:T2)  [unwired: 2 in, 2 out]
                n247 = Unbundle By Name(w614) -> ("Left"=w613:i32, "Top"=w612:i32)
                n248 = Subtract(x=w613, y=20) -> (x-y=w593:i32)
                n249 = Subtract(x=w612, y=76) -> (x-y=w592:i32)
                n250 = Bundle By Name(cluster=w614, "Left"=w593, "Top"=w592) -> (w615:T2)
                n251 = Add(x=w593, y=20 ("Position:Left")) -> (x+y=w595:i32)
                n252 = Add(x=w592, y=10 ("Position:Top")) -> (x+y=w594:i32)
                n253 = property on="Pane" class="Pane"("Origin"=w615) -> ()  [unwired: 2 in, 2 out]
                n254 = property on="Choose file" class="Bool (strict)"("Left"=w595, "Top"=w594, "Height"=u32 65 ("Button Size:Height"), "Width"=u32 90 ("Button Size:Width")) -> ("Width"=w607:u32, "Left"=w606:i32, "Top"=w602:i32)  [unwired: 2 in, 2 out]
                n255 = Add(x=w602, y=25) -> (x+y=w600:i32)
                n256 = Compound Arithmetic op=ADD(w607, w606, 20 ("value")) -> (w605:u32)
                n257 = property on="Hold" class="Bool (strict)"("Left"=w605, "Top"=w600) -> ("Width"=w604:u32, "Left"=w603:i32, "Top"=w599:i32)  [unwired: 2 in, 2 out]
                n258 = Subtract(x=w599, y=22) -> (x-y=w580:i32)
                n259 = Compound Arithmetic op=ADD(w604, w603, 20 ("value")) -> (w582:u32)
                n260 = property on="Plot Selector" class="Ring (strict)"("Left"=w582, "Top"=w580, "Value"=w591) -> ("Width"=w581:u32)  [unwired: 2 in, 2 out]
                n261 = Compound Arithmetic op=ADD(w582, w581, u32 20 ("value")) -> (w590:u32)
                n262 = property on="Freq Lower Limit, Cur" class="DigNum (strict)"("Left"=w590, "Top"=w580) -> ("Width"=w583:u32)  [unwired: 2 in, 2 out]
                n263 = Compound Arithmetic op=ADD(w590, w583, u32 20 ("value")) -> (w588:u32)
                n264 = property on="Freq Upper Limit, Cur" class="DigNum (strict)"("Left"=w588, "Top"=w580) -> ("Width"=w586:u32)  [unwired: 2 in, 2 out]
                n265 = Compound Arithmetic op=ADD(w588, w586, u32 20 ("value")) -> (w587:u32)
                n266 = property on="Level Lower Limit, Cur" class="DigNum (strict)"("Left"=w587, "Top"=w580) -> ()  [unwired: 2 in, 2 out]
              }
              frame 6 {
                n267 = property on="Current Park Spectrum" class="WFGraph (strict)"() -> ("Position"=w652:T2)  [unwired: 2 in, 2 out]
                n268 = Unbundle By Name(w652) -> ("Left"=w651:i32, "Top"=w650:i32)
                n269 = Subtract(x=w651, y=20) -> (x-y=w631:i32)
                n270 = Subtract(x=w650, y=76) -> (x-y=w630:i32)
                n271 = Bundle By Name(cluster=w652, "Left"=w631, "Top"=w630) -> (w653:T2)
                n272 = Add(x=w631, y=20 ("Position:Left")) -> (x+y=w633:i32)
                n273 = Add(x=w630, y=10 ("Position:Top")) -> (x+y=w632:i32)
                n274 = property on="Pane" class="Pane"("Origin"=w653) -> ()  [unwired: 2 in, 2 out]
                n275 = property on="Choose file" class="Bool (strict)"("Left"=w633, "Top"=w632, "Height"=u32 65 ("Button Size:Height"), "Width"=u32 90 ("Button Size:Width")) -> ("Width"=w645:u32, "Left"=w644:i32, "Top"=w640:i32)  [unwired: 2 in, 2 out]
                n276 = Add(x=w640, y=25) -> (x+y=w638:i32)
                n277 = Compound Arithmetic op=ADD(w645, w644, 20 ("value")) -> (w643:u32)
                n278 = property on="Hold" class="Bool (strict)"("Left"=w643, "Top"=w638) -> ("Width"=w642:u32, "Left"=w641:i32, "Top"=w637:i32)  [unwired: 2 in, 2 out]
                n279 = Subtract(x=w637, y=22) -> (x-y=w618:i32)
                n280 = Compound Arithmetic op=ADD(w642, w641, 20 ("value")) -> (w620:u32)
                n281 = property on="Plot Selector" class="Ring (strict)"("Left"=w620, "Top"=w618, "Value"=w629) -> ("Width"=w619:u32)  [unwired: 2 in, 2 out]
                n282 = Compound Arithmetic op=ADD(w619, w620, u32 20 ("value")) -> (w628:u32)
                n283 = property on="Freq Lower Limit, Cur" class="DigNum (strict)"("Left"=w628, "Top"=w618) -> ("Width"=w621:u32)  [unwired: 2 in, 2 out]
                n284 = Compound Arithmetic op=ADD(w628, w621, u32 20 ("value")) -> (w626:u32)
                n285 = property on="Freq Upper Limit, Cur" class="DigNum (strict)"("Left"=w626, "Top"=w618) -> ("Width"=w624:u32)  [unwired: 2 in, 2 out]
                n286 = Compound Arithmetic op=ADD(w626, w624, u32 20 ("value")) -> (w625:u32)
                n287 = property on="Level Lower Limit, Cur" class="DigNum (strict)"("Left"=w625, "Top"=w618) -> ()  [unwired: 2 in, 2 out]
              }
              frame 7 {
                n288 = property on="Voltage Park Spectrum" class="WFGraph (strict)"() -> ("Position"=w690:T2)  [unwired: 2 in, 2 out]
                n289 = Unbundle By Name(w690) -> ("Left"=w689:i32, "Top"=w688:i32)
                n290 = Subtract(x=w689, y=20) -> (x-y=w671:i32)
                n291 = Subtract(x=w688, y=76) -> (x-y=w670:i32)
                n292 = Bundle By Name(cluster=w690, "Left"=w671, "Top"=w670) -> (w691:T2)
                n293 = Add(x=w671, y=20 ("Position:Left")) -> (x+y=w669:i32)
                n294 = Add(x=w670, y=10 ("Position:Top")) -> (x+y=w668:i32)
                n295 = property on="Pane" class="Pane"("Origin"=w691) -> ()  [unwired: 2 in, 2 out]
                n296 = property on="Choose file" class="Bool (strict)"("Left"=w669, "Top"=w668, "Height"=u32 65 ("Button Size:Height"), "Width"=u32 90 ("Button Size:Width")) -> ("Width"=w683:u32, "Left"=w682:i32, "Top"=w678:i32)  [unwired: 2 in, 2 out]
                n297 = Add(x=w678, y=25) -> (x+y=w676:i32)
                n298 = Compound Arithmetic op=ADD(w683, w682, 20 ("value")) -> (w681:u32)
                n299 = property on="Hold" class="Bool (strict)"("Left"=w681, "Top"=w676) -> ("Width"=w680:u32, "Left"=w679:i32, "Top"=w675:i32)  [unwired: 2 in, 2 out]
                n300 = Subtract(x=w675, y=22) -> (x-y=w656:i32)
                n301 = Compound Arithmetic op=ADD(w680, w679, 20 ("value")) -> (w657:u32)
                n302 = property on="Plot Selector" class="Ring (strict)"("Left"=w657, "Top"=w656, "Value"=w667) -> ("Width"=w658:u32)  [unwired: 2 in, 2 out]
                n303 = Compound Arithmetic op=ADD(w657, w658, u32 20 ("value")) -> (w666:u32)
                n304 = property on="Freq Lower Limit, Cur" class="DigNum (strict)"("Left"=w666, "Top"=w656) -> ("Width"=w662:u32)  [unwired: 2 in, 2 out]
                n305 = Compound Arithmetic op=ADD(w666, w662, u32 20 ("value")) -> (w665:u32)
                n306 = property on="Freq Upper Limit, Cur" class="DigNum (strict)"("Left"=w665, "Top"=w656) -> ("Width"=w663:u32)  [unwired: 2 in, 2 out]
                n307 = Compound Arithmetic op=ADD(w665, w663, u32 20 ("value")) -> (w664:u32)
                n308 = property on="Level Lower Limit, Cur" class="DigNum (strict)"("Left"=w664, "Top"=w656) -> ()  [unwired: 2 in, 2 out]
              }
            }
          }
        }
      }
      event "Plot Selector": Value Change {
        n309 = event-data() -> ("NewVal"=w694:u16)  [unwired: 1 in, 5 out]
        n310 = case shown="7" w694 {
          selector: w694 -> [_ w697 w724 w753 w782 w822 w860 w898 w936]
          frame Default {
          }
          frame 0 {
            n311 = property on="Current" class="WFGraph (strict)"() -> ("Position"=w720:T2)  [unwired: 2 in, 2 out]
            n312 = Unbundle By Name(w720) -> ("Left"=w719:i32, "Top"=w718:i32)
            n313 = Subtract(x=w719, y=20) -> (x-y=w699:i32)
            n314 = Subtract(x=w718, y=76) -> (x-y=w698:i32)
            n315 = Bundle By Name(cluster=w720, "Left"=w699, "Top"=w698) -> (w721:T2)
            n316 = Add(x=w699, y=20 ("Position:Left")) -> (x+y=w701:i32)
            n317 = Add(x=w698, y=10 ("Position:Top")) -> (x+y=w700:i32)
            n318 = property on="Pane" class="Pane"("Origin"=w721) -> ()  [unwired: 2 in, 2 out]
            n319 = property on="Choose file" class="Bool (strict)"("Left"=w701, "Top"=w700, "Height"=u32 65 ("Button Size:Height"), "Width"=u32 90 ("Button Size:Width")) -> ("Width"=w713:u32, "Left"=w712:i32, "Top"=w708:i32)  [unwired: 2 in, 2 out]
            n320 = Add(x=w708, y=25) -> (x+y=w706:i32)
            n321 = Compound Arithmetic op=ADD(w713, w712, 20 ("value")) -> (w711:u32)
            n322 = property on="Hold" class="Bool (strict)"("Left"=w711, "Top"=w706) -> ("Width"=w710:u32, "Left"=w709:i32, "Top"=w705:i32)  [unwired: 2 in, 2 out]
            n323 = Subtract(x=w705, y=22) -> (x-y=w696:i32)
            n324 = Compound Arithmetic op=ADD(w710, w709, 20 ("value")) -> (w695:u32)
            n325 = property on="Plot Selector" class="Ring (strict)"("Left"=w695, "Top"=w696, "Value"=w697) -> ()  [unwired: 2 in, 2 out]
          }
          frame 1 {
            n326 = property on="Voltage" class="WFGraph (strict)"() -> ("Position"=w749:T2)  [unwired: 2 in, 2 out]
            n327 = Unbundle By Name(w749) -> ("Left"=w748:i32, "Top"=w747:i32)
            n328 = Subtract(x=w748, y=20) -> (x-y=w726:i32)
            n329 = Subtract(x=w747, y=76) -> (x-y=w725:i32)
            n330 = Bundle By Name(cluster=w749, "Left"=w726, "Top"=w725) -> (w750:T2)
            n331 = Add(x=w726, y=20 ("Position:Left")) -> (x+y=w728:i32)
            n332 = Add(x=w725, y=10 ("Position:Top")) -> (x+y=w727:i32)
            n333 = property on="Pane" class="Pane"("Origin"=w750) -> ()  [unwired: 2 in, 2 out]
            n334 = property on="Choose file" class="Bool (strict)"("Left"=w728, "Top"=w727, "Height"=u32 65 ("Button Size:Height"), "Width"=u32 90 ("Button Size:Width")) -> ("Width"=w741:u32, "Left"=w740:i32, "Top"=w736:i32)  [unwired: 2 in, 2 out]
            n335 = Add(x=w736, y=25) -> (x+y=w734:i32)
            n336 = Compound Arithmetic op=ADD(w741, w740, 20 ("value")) -> (w739:u32)
            n337 = property on="Hold" class="Bool (strict)"("Left"=w739, "Top"=w734) -> ("Width"=w738:u32, "Left"=w737:i32, "Top"=w733:i32)  [unwired: 2 in, 2 out]
            n338 = Subtract(x=w733, y=22) -> (x-y=w731:i32)
            n339 = Compound Arithmetic op=ADD(w738, w737, 20 ("value")) -> (w745:u32)
            n340 = property on="Plot Selector" class="Ring (strict)"("Left"=w745, "Top"=w731, "Value"=w724) -> ()  [unwired: 2 in, 2 out]
          }
          frame 2 {
            n341 = property on="Current Godograph" class="XYGraph (strict)"() -> ("Position"=w778:T2)  [unwired: 2 in, 2 out]
            n342 = Unbundle By Name(w778) -> ("Left"=w777:i32, "Top"=w776:i32)
            n343 = Subtract(x=w777, y=20) -> (x-y=w755:i32)
            n344 = Subtract(x=w776, y=76) -> (x-y=w754:i32)
            n345 = Bundle By Name(cluster=w778, "Left"=w755, "Top"=w754) -> (w779:T2)
            n346 = Add(x=w755, y=20 ("Position:Left")) -> (x+y=w757:i32)
            n347 = Add(x=w754, y=10 ("Position:Top")) -> (x+y=w756:i32)
            n348 = property on="Pane" class="Pane"("Origin"=w779) -> ()  [unwired: 2 in, 2 out]
            n349 = property on="Choose file" class="Bool (strict)"("Left"=w757, "Top"=w756, "Height"=u32 65 ("Button Size:Height"), "Width"=u32 90 ("Button Size:Width")) -> ("Width"=w770:u32, "Left"=w769:i32, "Top"=w765:i32)  [unwired: 2 in, 2 out]
            n350 = Add(x=w765, y=25) -> (x+y=w763:i32)
            n351 = Compound Arithmetic op=ADD(w770, w769, 20 ("value")) -> (w768:u32)
            n352 = property on="Hold" class="Bool (strict)"("Left"=w768, "Top"=w763) -> ("Width"=w767:u32, "Left"=w766:i32, "Top"=w762:i32)  [unwired: 2 in, 2 out]
            n353 = Subtract(x=w762, y=22) -> (x-y=w760:i32)
            n354 = Compound Arithmetic op=ADD(w767, w766, 20 ("value")) -> (w774:u32)
            n355 = property on="Plot Selector" class="Ring (strict)"("Left"=w774, "Top"=w760, "Value"=w753) -> ()  [unwired: 2 in, 2 out]
          }
          frame 3 {
            n356 = property on="Voltage Godograph" class="XYGraph (strict)"() -> ("Position"=w809:T2)  [unwired: 2 in, 2 out]
            n357 = Unbundle By Name(w809) -> ("Left"=w808:i32, "Top"=w807:i32)
            n358 = Subtract(x=w808, y=20) -> (x-y=w784:i32)
            n359 = Subtract(x=w807, y=76) -> (x-y=w783:i32)
            n360 = Bundle By Name(cluster=w809, "Left"=w784, "Top"=w783) -> (w810:T2)
            n361 = Add(x=w784, y=20 ("Position:Left")) -> (x+y=w786:i32)
            n362 = Add(x=w783, y=10 ("Position:Top")) -> (x+y=w785:i32)
            n363 = property on="Pane" class="Pane"("Origin"=w810) -> ()  [unwired: 2 in, 2 out]
            n364 = property on="Choose file" class="Bool (strict)"("Left"=w786, "Top"=w785, "Height"=u32 65 ("Button Size:Height"), "Width"=u32 90 ("Button Size:Width")) -> ("Width"=w799:u32, "Left"=w798:i32, "Top"=w794:i32)  [unwired: 2 in, 2 out]
            n365 = Add(x=w794, y=25) -> (x+y=w792:i32)
            n366 = Compound Arithmetic op=ADD(w799, w798, 20 ("value")) -> (w797:u32)
            n367 = property on="Hold" class="Bool (strict)"("Left"=w797, "Top"=w792) -> ("Width"=w796:u32, "Left"=w795:i32, "Top"=w791:i32)  [unwired: 2 in, 2 out]
            n368 = Subtract(x=w791, y=22) -> (x-y=w789:i32)
            n369 = Compound Arithmetic op=ADD(w796, w795, 20 ("value")) -> (w803:u32)
            n370 = property on="Plot Selector" class="Ring (strict)"("Left"=w803, "Top"=w789, "Value"=w782) -> ()  [unwired: 2 in, 2 out]
          }
          frame 4 {
            n371 = property on="Current Spectrum" class="WFGraph (strict)"() -> ("Position"=w845:T2)  [unwired: 2 in, 2 out]
            n372 = Unbundle By Name(w845) -> ("Left"=w844:i32, "Top"=w843:i32)
            n373 = Subtract(x=w844, y=20) -> (x-y=w824:i32)
            n374 = Subtract(x=w843, y=76) -> (x-y=w823:i32)
            n375 = Bundle By Name(cluster=w845, "Left"=w824, "Top"=w823) -> (w846:T2)
            n376 = Add(x=w824, y=20 ("Position:Left")) -> (x+y=w826:i32)
            n377 = Add(x=w823, y=10 ("Position:Top")) -> (x+y=w825:i32)
            n378 = property on="Pane" class="Pane"("Origin"=w846) -> ()  [unwired: 2 in, 2 out]
            n379 = property on="Choose file" class="Bool (strict)"("Left"=w826, "Top"=w825, "Height"=u32 65 ("Button Size:Height"), "Width"=u32 90 ("Button Size:Width")) -> ("Width"=w838:u32, "Left"=w837:i32, "Top"=w833:i32)  [unwired: 2 in, 2 out]
            n380 = Add(x=w833, y=25) -> (x+y=w831:i32)
            n381 = Compound Arithmetic op=ADD(w838, w837, 20 ("value")) -> (w836:u32)
            n382 = property on="Hold" class="Bool (strict)"("Left"=w836, "Top"=w831) -> ("Width"=w835:u32, "Left"=w834:i32, "Top"=w830:i32)  [unwired: 2 in, 2 out]
            n383 = Subtract(x=w830, y=22) -> (x-y=w811:i32)
            n384 = Compound Arithmetic op=ADD(w835, w834, 20 ("value")) -> (w812:u32)
            n385 = property on="Plot Selector" class="Ring (strict)"("Left"=w812, "Top"=w811, "Value"=w822) -> ("Width"=w813:u32)  [unwired: 2 in, 2 out]
            n386 = Compound Arithmetic op=ADD(w812, w813, u32 20 ("value")) -> (w821:u32)
            n387 = property on="Freq Lower Limit, Cur" class="DigNum (strict)"("Left"=w821, "Top"=w811) -> ("Width"=w814:u32)  [unwired: 2 in, 2 out]
            n388 = Compound Arithmetic op=ADD(w821, w814, u32 20 ("value")) -> (w819:u32)
            n389 = property on="Freq Upper Limit, Cur" class="DigNum (strict)"("Left"=w819, "Top"=w811) -> ("Width"=w817:u32)  [unwired: 2 in, 2 out]
            n390 = Compound Arithmetic op=ADD(w819, w817, u32 20 ("value")) -> (w818:u32)
            n391 = property on="Level Lower Limit, Cur" class="DigNum (strict)"("Left"=w818, "Top"=w811) -> ()  [unwired: 2 in, 2 out]
          }
          frame 5 {
            n392 = property on="Voltage Spectrum" class="WFGraph (strict)"() -> ("Position"=w883:T2)  [unwired: 2 in, 2 out]
            n393 = Unbundle By Name(w883) -> ("Left"=w882:i32, "Top"=w881:i32)
            n394 = Subtract(x=w882, y=20) -> (x-y=w862:i32)
            n395 = Subtract(x=w881, y=76) -> (x-y=w861:i32)
            n396 = Bundle By Name(cluster=w883, "Left"=w862, "Top"=w861) -> (w884:T2)
            n397 = Add(x=w862, y=20 ("Position:Left")) -> (x+y=w864:i32)
            n398 = Add(x=w861, y=10 ("Position:Top")) -> (x+y=w863:i32)
            n399 = property on="Pane" class="Pane"("Origin"=w884) -> ()  [unwired: 2 in, 2 out]
            n400 = property on="Choose file" class="Bool (strict)"("Left"=w864, "Top"=w863, "Height"=u32 65 ("Button Size:Height"), "Width"=u32 90 ("Button Size:Width")) -> ("Width"=w876:u32, "Left"=w875:i32, "Top"=w871:i32)  [unwired: 2 in, 2 out]
            n401 = Add(x=w871, y=25) -> (x+y=w869:i32)
            n402 = Compound Arithmetic op=ADD(w876, w875, 20 ("value")) -> (w874:u32)
            n403 = property on="Hold" class="Bool (strict)"("Left"=w874, "Top"=w869) -> ("Width"=w873:u32, "Left"=w872:i32, "Top"=w868:i32)  [unwired: 2 in, 2 out]
            n404 = Subtract(x=w868, y=22) -> (x-y=w849:i32)
            n405 = Compound Arithmetic op=ADD(w873, w872, 20 ("value")) -> (w851:u32)
            n406 = property on="Plot Selector" class="Ring (strict)"("Left"=w851, "Top"=w849, "Value"=w860) -> ("Width"=w850:u32)  [unwired: 2 in, 2 out]
            n407 = Compound Arithmetic op=ADD(w851, w850, u32 20 ("value")) -> (w859:u32)
            n408 = property on="Freq Lower Limit, Cur" class="DigNum (strict)"("Left"=w859, "Top"=w849) -> ("Width"=w852:u32)  [unwired: 2 in, 2 out]
            n409 = Compound Arithmetic op=ADD(w859, w852, u32 20 ("value")) -> (w857:u32)
            n410 = property on="Freq Upper Limit, Cur" class="DigNum (strict)"("Left"=w857, "Top"=w849) -> ("Width"=w855:u32)  [unwired: 2 in, 2 out]
            n411 = Compound Arithmetic op=ADD(w857, w855, u32 20 ("value")) -> (w856:u32)
            n412 = property on="Level Lower Limit, Cur" class="DigNum (strict)"("Left"=w856, "Top"=w849) -> ()  [unwired: 2 in, 2 out]
          }
          frame 6 {
            n413 = property on="Current Park Spectrum" class="WFGraph (strict)"() -> ("Position"=w921:T2)  [unwired: 2 in, 2 out]
            n414 = Unbundle By Name(w921) -> ("Left"=w920:i32, "Top"=w919:i32)
            n415 = Subtract(x=w920, y=20) -> (x-y=w900:i32)
            n416 = Subtract(x=w919, y=76) -> (x-y=w899:i32)
            n417 = Bundle By Name(cluster=w921, "Left"=w900, "Top"=w899) -> (w922:T2)
            n418 = Add(x=w900, y=20 ("Position:Left")) -> (x+y=w902:i32)
            n419 = Add(x=w899, y=10 ("Position:Top")) -> (x+y=w901:i32)
            n420 = property on="Pane" class="Pane"("Origin"=w922) -> ()  [unwired: 2 in, 2 out]
            n421 = property on="Choose file" class="Bool (strict)"("Left"=w902, "Top"=w901, "Height"=u32 65 ("Button Size:Height"), "Width"=u32 90 ("Button Size:Width")) -> ("Width"=w914:u32, "Left"=w913:i32, "Top"=w909:i32)  [unwired: 2 in, 2 out]
            n422 = Add(x=w909, y=25) -> (x+y=w907:i32)
            n423 = Compound Arithmetic op=ADD(w914, w913, 20 ("value")) -> (w912:u32)
            n424 = property on="Hold" class="Bool (strict)"("Left"=w912, "Top"=w907) -> ("Width"=w911:u32, "Left"=w910:i32, "Top"=w906:i32)  [unwired: 2 in, 2 out]
            n425 = Subtract(x=w906, y=22) -> (x-y=w887:i32)
            n426 = Compound Arithmetic op=ADD(w911, w910, 20 ("value")) -> (w889:u32)
            n427 = property on="Plot Selector" class="Ring (strict)"("Left"=w889, "Top"=w887, "Value"=w898) -> ("Width"=w888:u32)  [unwired: 2 in, 2 out]
            n428 = Compound Arithmetic op=ADD(w888, w889, u32 20 ("value")) -> (w897:u32)
            n429 = property on="Freq Lower Limit, Cur" class="DigNum (strict)"("Left"=w897, "Top"=w887) -> ("Width"=w890:u32)  [unwired: 2 in, 2 out]
            n430 = Compound Arithmetic op=ADD(w897, w890, u32 20 ("value")) -> (w895:u32)
            n431 = property on="Freq Upper Limit, Cur" class="DigNum (strict)"("Left"=w895, "Top"=w887) -> ("Width"=w893:u32)  [unwired: 2 in, 2 out]
            n432 = Compound Arithmetic op=ADD(w895, w893, u32 20 ("value")) -> (w894:u32)
            n433 = property on="Level Lower Limit, Cur" class="DigNum (strict)"("Left"=w894, "Top"=w887) -> ()  [unwired: 2 in, 2 out]
          }
          frame 7 {
            n434 = property on="Voltage Park Spectrum" class="WFGraph (strict)"() -> ("Position"=w959:T2)  [unwired: 2 in, 2 out]
            n435 = Unbundle By Name(w959) -> ("Left"=w958:i32, "Top"=w957:i32)
            n436 = Subtract(x=w958, y=20) -> (x-y=w940:i32)
            n437 = Subtract(x=w957, y=76) -> (x-y=w939:i32)
            n438 = Bundle By Name(cluster=w959, "Left"=w940, "Top"=w939) -> (w960:T2)
            n439 = Add(x=w940, y=20 ("Position:Left")) -> (x+y=w938:i32)
            n440 = Add(x=w939, y=10 ("Position:Top")) -> (x+y=w937:i32)
            n441 = property on="Pane" class="Pane"("Origin"=w960) -> ()  [unwired: 2 in, 2 out]
            n442 = property on="Choose file" class="Bool (strict)"("Left"=w938, "Top"=w937, "Height"=u32 65 ("Button Size:Height"), "Width"=u32 90 ("Button Size:Width")) -> ("Width"=w952:u32, "Left"=w951:i32, "Top"=w947:i32)  [unwired: 2 in, 2 out]
            n443 = Add(x=w947, y=25) -> (x+y=w945:i32)
            n444 = Compound Arithmetic op=ADD(w952, w951, 20 ("value")) -> (w950:u32)
            n445 = property on="Hold" class="Bool (strict)"("Left"=w950, "Top"=w945) -> ("Width"=w949:u32, "Left"=w948:i32, "Top"=w944:i32)  [unwired: 2 in, 2 out]
            n446 = Subtract(x=w944, y=22) -> (x-y=w925:i32)
            n447 = Compound Arithmetic op=ADD(w949, w948, 20 ("value")) -> (w926:u32)
            n448 = property on="Plot Selector" class="Ring (strict)"("Left"=w926, "Top"=w925, "Value"=w936) -> ("Width"=w927:u32)  [unwired: 2 in, 2 out]
            n449 = Compound Arithmetic op=ADD(w926, w927, u32 20 ("value")) -> (w935:u32)
            n450 = property on="Freq Lower Limit, Cur" class="DigNum (strict)"("Left"=w935, "Top"=w925) -> ("Width"=w931:u32)  [unwired: 2 in, 2 out]
            n451 = Compound Arithmetic op=ADD(w935, w931, u32 20 ("value")) -> (w934:u32)
            n452 = property on="Freq Upper Limit, Cur" class="DigNum (strict)"("Left"=w934, "Top"=w925) -> ("Width"=w932:u32)  [unwired: 2 in, 2 out]
            n453 = Compound Arithmetic op=ADD(w934, w932, u32 20 ("value")) -> (w933:u32)
            n454 = property on="Level Lower Limit, Cur" class="DigNum (strict)"("Left"=w933, "Top"=w925) -> ()  [unwired: 2 in, 2 out]
          }
        }
      }
      event "Current Amplitude Range": Value Change {
        n455 = event-data() -> ("NewVal"=w963:dbl)  [unwired: 1 in]
        n456 = Negate(x=w963) -> (-x=w964:dbl)
        n457 = property on="Current" class="WFGraph (strict)"("YScale.Maximum"=w963, "YScale.Minimum"=w964) -> ()  [unwired: 2 in, 2 out]
      }
      event "Voltage Amplitude Range": Value Change {
        n458 = event-data() -> ("NewVal"=w965:dbl)  [unwired: 1 in]
        n459 = Negate(x=w965) -> (-x=w966:dbl)
        n460 = property on="Voltage" class="WFGraph (strict)"("YScale.Maximum"=w965, "YScale.Minimum"=w966) -> ()  [unwired: 2 in, 2 out]
      }
      event "Current Godograph Range": Value Change {
        n461 = event-data() -> ("NewVal"=w968:dbl)  [unwired: 1 in]
        n462 = Negate(x=w968) -> (-x=w967:dbl)
        n463 = property on="Current Godograph" class="XYGraph (strict)"("YScale.Maximum"=w968, "YScale.Minimum"=w967, "XScale.Maximum"=w968, "XScale.Minimum"=w967) -> ()  [unwired: 2 in, 2 out]
      }
      event "Voltage Godograph Range": Value Change {
        n464 = event-data() -> ("NewVal"=w969:dbl)  [unwired: 1 in]
        n465 = Negate(x=w969) -> (-x=w970:dbl)
        n466 = property on="Current Godograph" class="XYGraph (strict)"("YScale.Maximum"=w969, "YScale.Minimum"=w970, "XScale.Maximum"=w969, "XScale.Minimum"=w970) -> ()  [unwired: 2 in, 2 out]
      }
      event "Freq Lower Limit, Cur": Value Change {
        n467 = event-data() -> ("NewVal"=w971:dbl)  [unwired: 1 in]
        n468 = flat-sequence {
          tunnel: w971 -> [w976]
          frame #0 {
            n469 = property on="Freq Upper Limit, Cur" class="DigNum (strict)"() -> ("Value"=w975:dbl)  [unwired: 2 in, 2 out]
            n470 = Subtract(x=w975, y=10.0) -> (x-y=w972:dbl)
            n471 = Greater?(x=w976, y=w972) -> (0:w973:bool)
            n472 = case shown="True" w973 {
              tunnel: w972 -> [_ w977]
              frame False {
              }
              frame True {
                n473 = property on="Freq Lower Limit, Cur" class="DigNum (strict)"("Value"=w977) -> ()  [unwired: 2 in, 2 out]
              }
            }
          }
          frame #1 {
            n474 = property on="Freq Lower Limit, Cur" class="DigNum (strict)"() -> ("Value"=w978:dbl)  [unwired: 2 in, 2 out]
            n475 = property on="Current Spectrum" class="WFGraph (strict)"("XScale.Minimum"=w978) -> ()  [unwired: 2 in, 2 out]
            n476 = property on="Voltage Spectrum" class="WFGraph (strict)"("XScale.Minimum"=w978) -> ()  [unwired: 2 in, 2 out]
            n477 = property on="Current Park Spectrum" class="WFGraph (strict)"("XScale.Minimum"=w978) -> ()  [unwired: 2 in, 2 out]
            n478 = property on="Voltage Park Spectrum" class="WFGraph (strict)"("XScale.Minimum"=w978) -> ()  [unwired: 2 in, 2 out]
          }
        }
      }
      event "Freq Upper Limit, Cur": Value Change {
        n479 = event-data() -> ("NewVal"=w979:dbl)  [unwired: 1 in]
        n480 = flat-sequence {
          tunnel: w979 -> [w984]
          frame #0 {
            n481 = property on="Freq Lower Limit, Cur" class="DigNum (strict)"() -> ("Value"=w983:dbl)  [unwired: 2 in, 2 out]
            n482 = Add(x=w983, y=10.0) -> (x+y=w980:dbl)
            n483 = Less?(x=w984, y=w980) -> (x < y?=w981:bool)
            n484 = case shown="True" w981 {
              tunnel: w980 -> [_ w985]
              frame False {
              }
              frame True {
                n485 = property on="Freq Upper Limit, Cur" class="DigNum (strict)"("Value"=w985) -> ()  [unwired: 2 in, 2 out]
              }
            }
          }
          frame #1 {
            n486 = property on="Freq Upper Limit, Cur" class="DigNum (strict)"() -> ("Value"=w986:dbl)  [unwired: 2 in, 2 out]
            n487 = property on="Current Spectrum" class="WFGraph (strict)"("XScale.Maximum"=w986) -> ()  [unwired: 2 in, 2 out]
            n488 = property on="Voltage Spectrum" class="WFGraph (strict)"("XScale.Maximum"=w986) -> ()  [unwired: 2 in, 2 out]
            n489 = property on="Current Park Spectrum" class="WFGraph (strict)"("XScale.Maximum"=w986) -> ()  [unwired: 2 in, 2 out]
            n490 = property on="Voltage Park Spectrum" class="WFGraph (strict)"("XScale.Maximum"=w986) -> ()  [unwired: 2 in, 2 out]
          }
        }
      }
      event "Level Lower Limit, Cur": Value Change {
        n491 = event-data() -> ("NewVal"=w987:dbl)  [unwired: 1 in]
        n492 = flat-sequence {
          tunnel: [w988] -> _
          tunnel: w987 -> [w988]
          frame #0 {
            w990 = -10.0 ("y")
            n493 = Greater?(x=w988, y=w990) -> (0:w991:bool)
            n494 = Select(t=w990, s=w991, f=w988) -> (s? t:f=w989:dbl)
            n495 = property on="Level Lower Limit, Cur" class="DigNum (strict)"("Value"=w989) -> ()  [unwired: 2 in, 2 out]
          }
          frame #1 {
            n496 = property on="Level Lower Limit, Cur" class="DigNum (strict)"() -> ("Value"=w992:dbl)  [unwired: 2 in, 2 out]
            n497 = property on="Current Spectrum" class="WFGraph (strict)"("YScale.Minimum"=w992) -> ()  [unwired: 2 in, 2 out]
            n498 = property on="Voltage Spectrum" class="WFGraph (strict)"("YScale.Minimum"=w992) -> ()  [unwired: 2 in, 2 out]
            n499 = property on="Current Park Spectrum" class="WFGraph (strict)"("YScale.Minimum"=w992) -> ()  [unwired: 2 in, 2 out]
            n500 = property on="Voltage Park Spectrum" class="WFGraph (strict)"("YScale.Minimum"=w992) -> ()  [unwired: 2 in, 2 out]
          }
        }
      }
    }
  }
  n501 = while {
    tunnel: w1 -> [w995]
    stop <- FALSE stop-if-true
    n502 = Dequeue Element(queue=w995) -> (element=w993:path)  [unwired: 2 in, 3 out]
    n503 = flat-sequence {
      tunnel: w993 -> [w1016]
      frame #0 {
        n504 = TDMS Open(5:FALSE ("create index file? (T)"), 11:w1016) -> (3:w1013:refnum<k34>)  [unwired: 5 in, 1 out]
        n505 = TDMS Read(0:w1013, 5:"Time-Domain" ("group name in"), 7:string[] ["Ua", "Ub", "Uc", "Ud", "Uq", "Ia", "Ib", "Ic", "Id", "Iq"] ("channel name(s) in")) -> (10:w1025:waveform(dbl)[])  [unwired: 5 in, 5 out]
        n506 = TDMS Read(0:w1013, 5:"Frequency-Domain" ("group name in"), 7:string[] ["Ua", "Ub", "Uc", "Ia", "Ib", "Ic", "U_Park", "I_Park"] ("channel name(s) in")) -> (10:w1021:waveform(dbl)[])  [unwired: 5 in, 5 out]
        n507 = Index Array(array=w1025, index #1=4 ("index"), index #2=3 ("index")) -> (element #1=w1035:waveform(dbl), element #2=w1033:waveform(dbl))
        n508 = Index Array(array=w1025, index #1=9 ("index"), index #2=8 ("index")) -> (element #1=w1028:waveform(dbl), element #2=w1030:waveform(dbl))
        n509 = Array Subset(array=w1025, index=0, length=3) -> (w1010:waveform(dbl)[])
        n510 = Array Subset(array=w1025, index=5, length=3) -> (w1012:waveform(dbl)[])
        n511 = Unbundle By Name(w1035) -> ("Y"=w1034:dbl[])
        n512 = Unbundle By Name(w1033) -> ("Y"=w1032:dbl[])
        n513 = Unbundle By Name(w1028) -> ("Y"=w1029:dbl[])
        n514 = Unbundle By Name(w1030) -> ("Y"=w1031:dbl[])
        n515 = Array Subset(array=w1021, index=3, length=3) -> (w1006:waveform(dbl)[])
        n516 = Index Array(array=w1021, index #1=6 ("index"), index #2=7 ("index")) -> (element #1=w1004:waveform(dbl), element #2=w1002:waveform(dbl))
        n517 = Array Subset(array=w1021, index=0, length=3) -> (w1008:waveform(dbl)[])
        n518 = case shown="True" "Hold" {
          tunnel: w1010 -> [w1072 w1075]
          tunnel: [w1072 w1073] -> w1009
          frame False {
          }
          frame True {
            n519 = property on="Voltage store" class="Arr (strict)"() -> ("Value"=w1074:waveform(dbl)[])  [unwired: 2 in, 2 out]
            n520 = Insert Into Array(array=w1074, new element=w1075) -> (w1073:waveform(dbl)[])  [unwired: 1 in]
          }
        }
        "Voltage" <- w1009
        "Voltage store" <- w1009
        n521 = case shown="True" "Hold" {
          tunnel: w1012 -> [w1076 w1079]
          tunnel: [w1076 w1077] -> w1011
          frame False {
          }
          frame True {
            n522 = property on="Current store" class="Arr (strict)"() -> ("Value"=w1078:waveform(dbl)[])  [unwired: 2 in, 2 out]
            n523 = Insert Into Array(array=w1078, new element=w1079) -> (w1077:waveform(dbl)[])  [unwired: 1 in]
          }
        }
        "Current" <- w1011
        "Current store" <- w1011
        n524 = case shown="True" "Hold" {
          tunnel: [w1064 w1066] -> w1005
          tunnel: w1006 -> [w1064 w1065]
          frame False {
          }
          frame True {
            n525 = property on="Current Spectrum store" class="Arr (strict)"() -> ("Value"=w1067:waveform(dbl)[])  [unwired: 2 in, 2 out]
            n526 = Insert Into Array(array=w1067, new element=w1065) -> (w1066:waveform(dbl)[])  [unwired: 1 in]
          }
        }
        "Current Spectrum" <- w1005
        "Current Spectrum store" <- w1005
        n527 = case shown="True" "Hold" {
          tunnel: [w1060 w1062] -> w1003
          tunnel: w1004 -> [w1059 w1061]
          frame False {
            n528 = Build Array(w1059) -> (w1060:waveform(dbl)[])
          }
          frame True {
            n529 = property on="Voltage Park Spectrum store" class="Arr (strict)"() -> ("Value"=w1063:waveform(dbl)[])  [unwired: 2 in, 2 out]
            n530 = Insert Into Array(array=w1063, new element=w1061) -> (w1062:waveform(dbl)[])  [unwired: 1 in]
          }
        }
        "Voltage Park Spectrum" <- w1003
        "Voltage Park Spectrum store" <- w1003
        n531 = case shown="True" "Hold" {
          tunnel: [w1055 w1057] -> w1001
          tunnel: w1002 -> [w1054 w1056]
          frame False {
            n532 = Build Array(w1054) -> (w1055:waveform(dbl)[])
          }
          frame True {
            n533 = property on="Current Park Spectrum store" class="Arr (strict)"() -> ("Value"=w1058:waveform(dbl)[])  [unwired: 2 in, 2 out]
            n534 = Insert Into Array(array=w1058, new element=w1056) -> (w1057:waveform(dbl)[])  [unwired: 1 in]
          }
        }
        "Current Park Spectrum" <- w1001
        "Current Park Spectrum store" <- w1001
        n535 = case shown="True" "Hold" {
          tunnel: [w1068 w1070] -> w1007
          tunnel: w1008 -> [w1068 w1069]
          frame False {
          }
          frame True {
            n536 = property on="Voltage Spectrum store" class="Arr (strict)"() -> ("Value"=w1071:waveform(dbl)[])  [unwired: 2 in, 2 out]
            n537 = Insert Into Array(array=w1071, new element=w1069) -> (w1070:waveform(dbl)[])  [unwired: 1 in]
          }
        }
        "Voltage Spectrum" <- w1007
        "Voltage Spectrum store" <- w1007
        n538 = Bundle("Y"=w1034, "Y"=w1032) -> (w1000:cluster{"Y":dbl[], "Y":dbl[]})  [unwired: 1 in]
        n539 = Bundle("Y"=w1029, "Y"=w1031) -> (w997:cluster{"Y":dbl[], "Y":dbl[]})  [unwired: 1 in]
        n540 = case shown="True" "Hold" {
          tunnel: w1000 -> [w1050 w1053]
          tunnel: [w1049 w1051] -> w999
          frame False {
            n541 = Build Array(w1050) -> (w1049:cluster{"Y":dbl[], "Y":dbl[]}[])
          }
          frame True {
            n542 = property on="Voltage Godograph store" class="Arr (strict)"() -> ("Value"=w1052:cluster{"Y":dbl[], "Y":dbl[]}[])  [unwired: 2 in, 2 out]
            n543 = Insert Into Array(array=w1052, new element=w1053) -> (w1051:cluster{"Y":dbl[], "Y":dbl[]}[])  [unwired: 1 in]
          }
        }
        "Voltage Godograph" <- w999
        "Voltage Godograph store" <- w999
        n544 = case shown="True" "Hold" {
          tunnel: w997 -> [w1045 w1048]
          tunnel: [w1044 w1046] -> w998
          frame False {
            n545 = Build Array(w1045) -> (w1044:cluster{"Y":dbl[], "Y":dbl[]}[])
          }
          frame True {
            n546 = property on="Current Godograph store" class="Arr (strict)"() -> ("Value"=w1047:cluster{"Y":dbl[], "Y":dbl[]}[])  [unwired: 2 in, 2 out]
            n547 = Insert Into Array(array=w1047, new element=w1048) -> (w1046:cluster{"Y":dbl[], "Y":dbl[]}[])  [unwired: 1 in]
          }
        }
        "Current Godograph" <- w998
        "Current Godograph store" <- w998
      }
    }
  }
